vi "BRig_RT__Case_Exp__State_initTrial__v17.vi"(0 "input_dataCurrent":u16[](array[numeric]), 9 "input_dataBlock":u16[][](array[numeric]), 11 "input_dataTrial":u16[][](array[numeric]), 12 "input_dataExp":u16[](array[numeric])) -> (1 "output_iTrial":u16, 2 "output_nTrial":u16, 3 "output_SolenoidReward":bool, 4 "output_dataCurrent":u16[](array[numeric]), 10 "output_dataBlock":u16[][](array[numeric]), 15 "output_dataTrial":u16[][](array[numeric]))   [LabVIEW 2014]
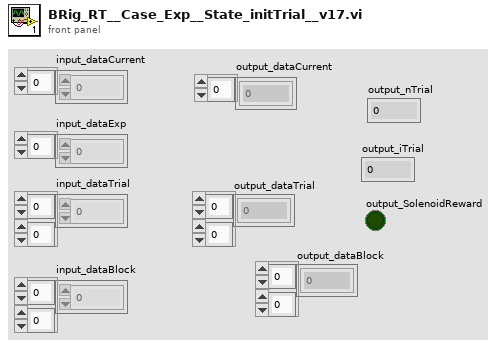
[diagram p1: front panel]
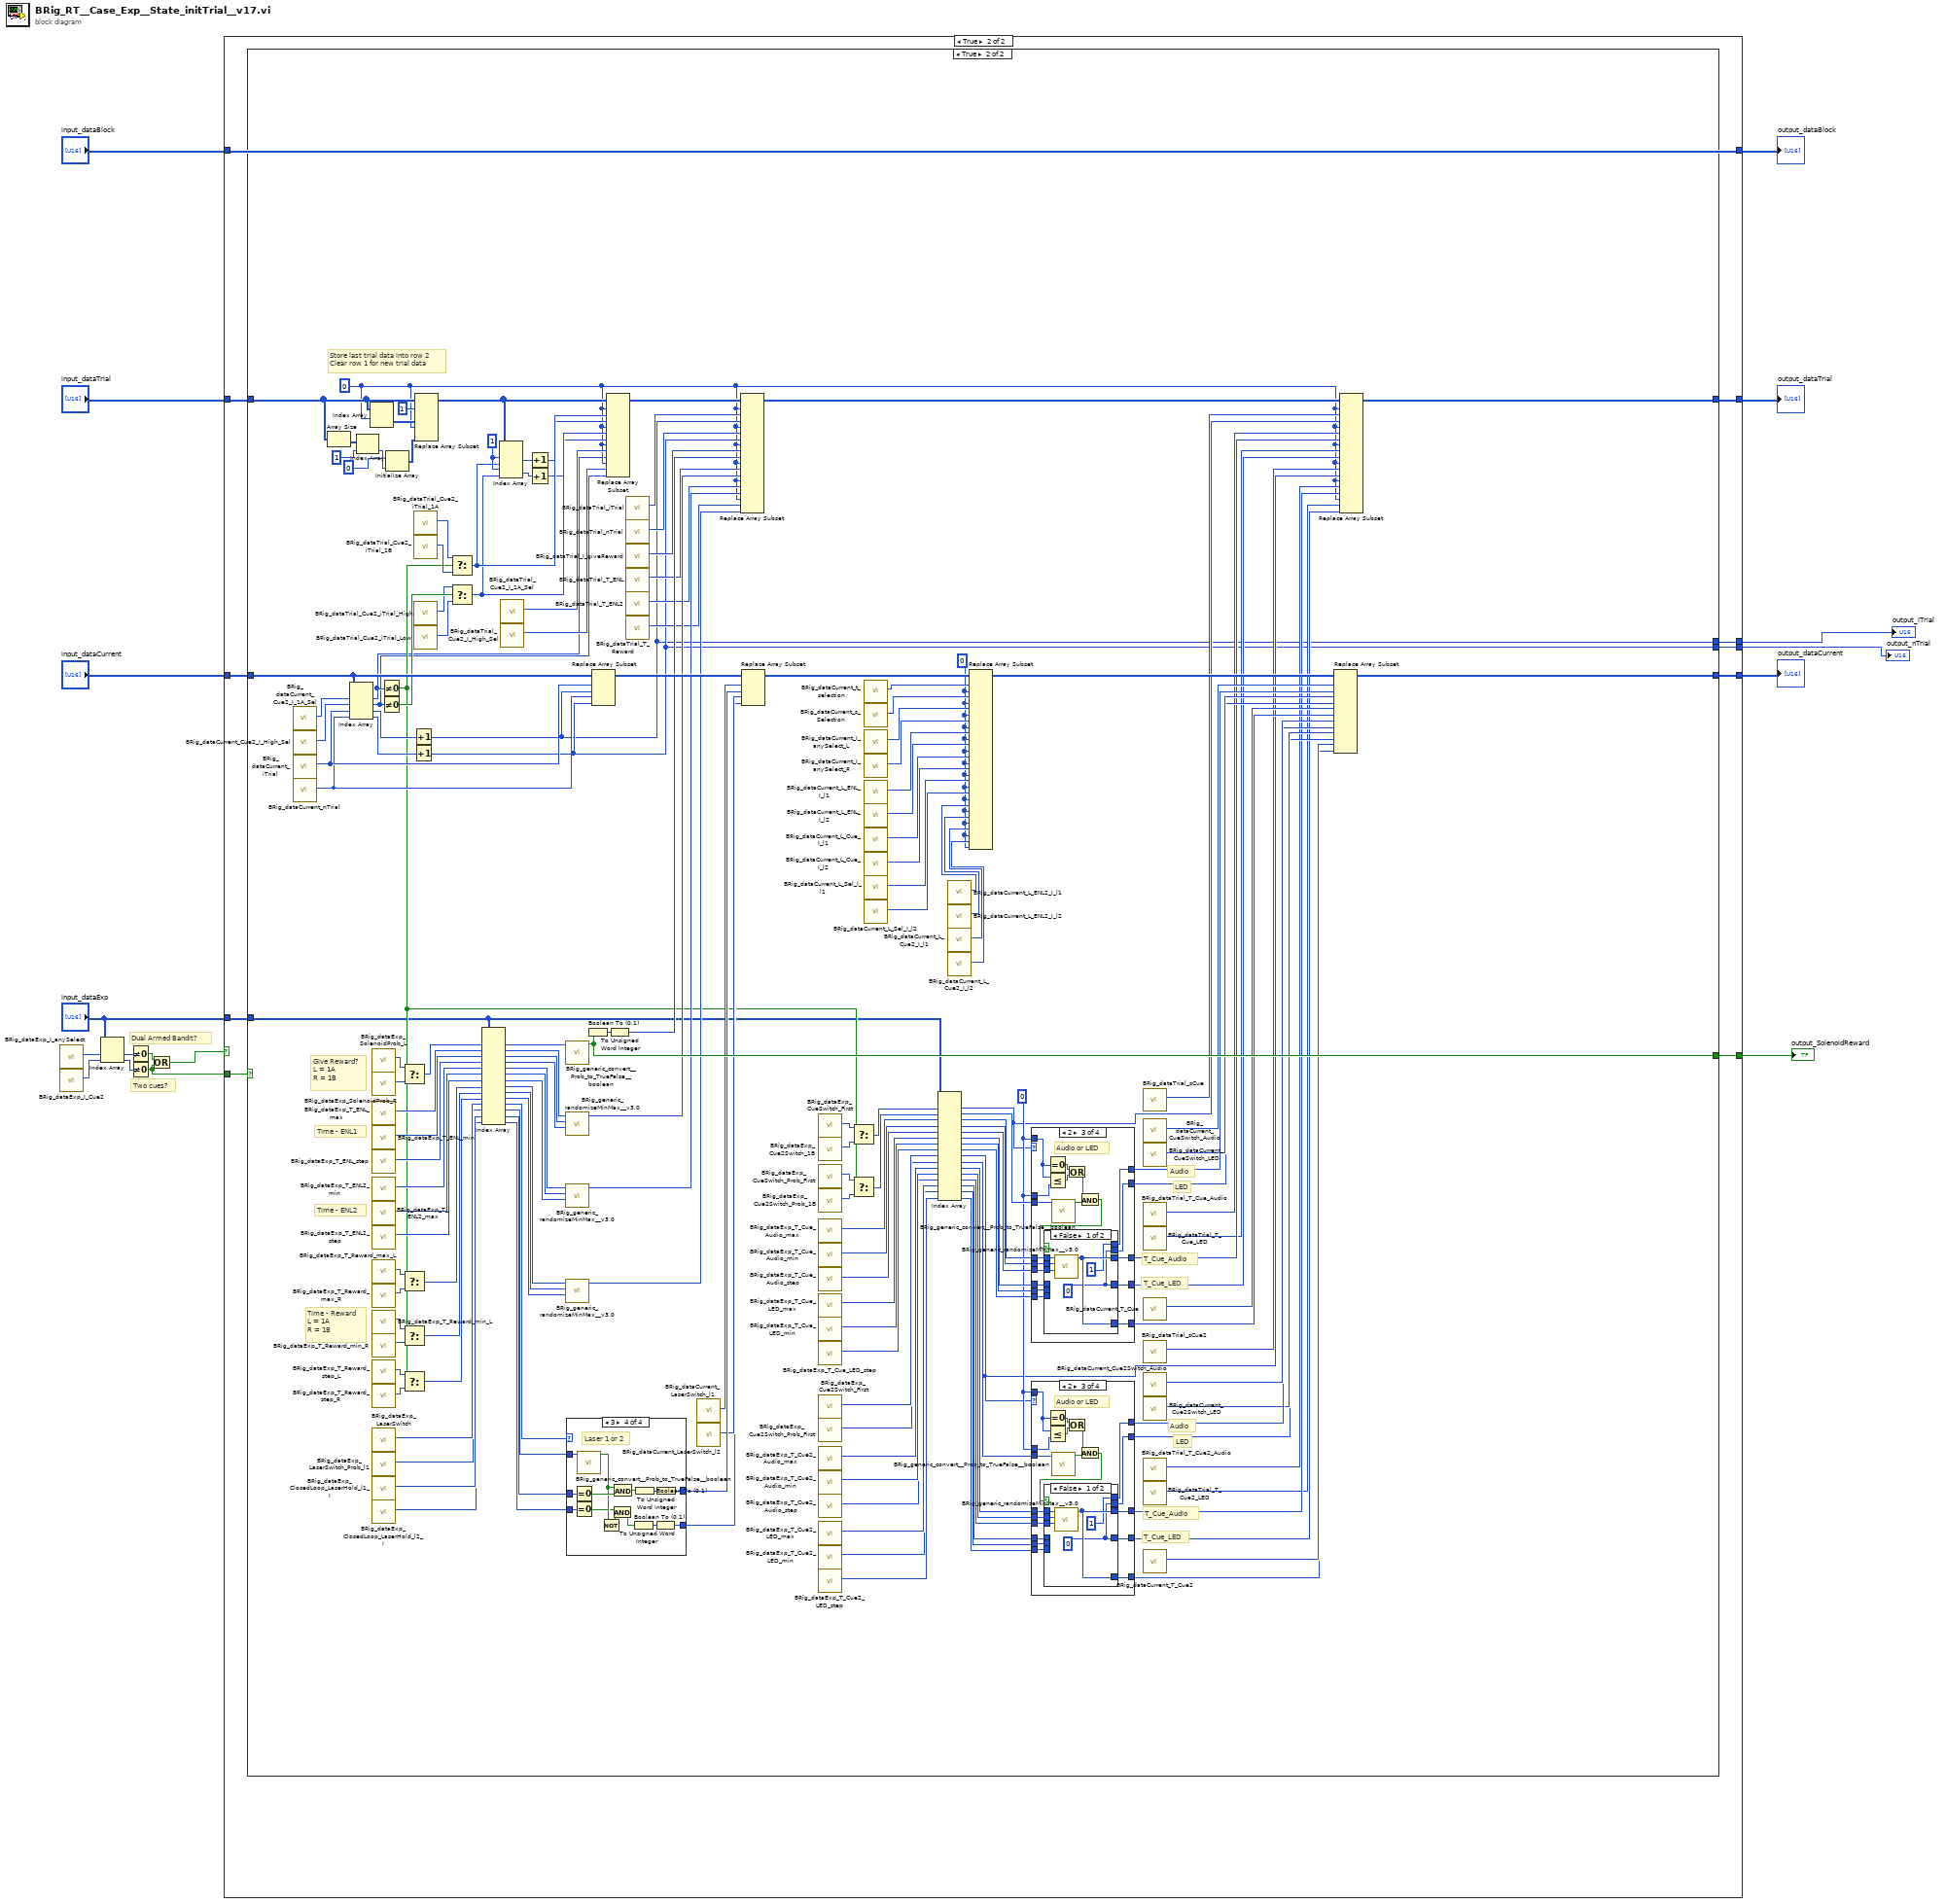
[diagram p0: block diagram]
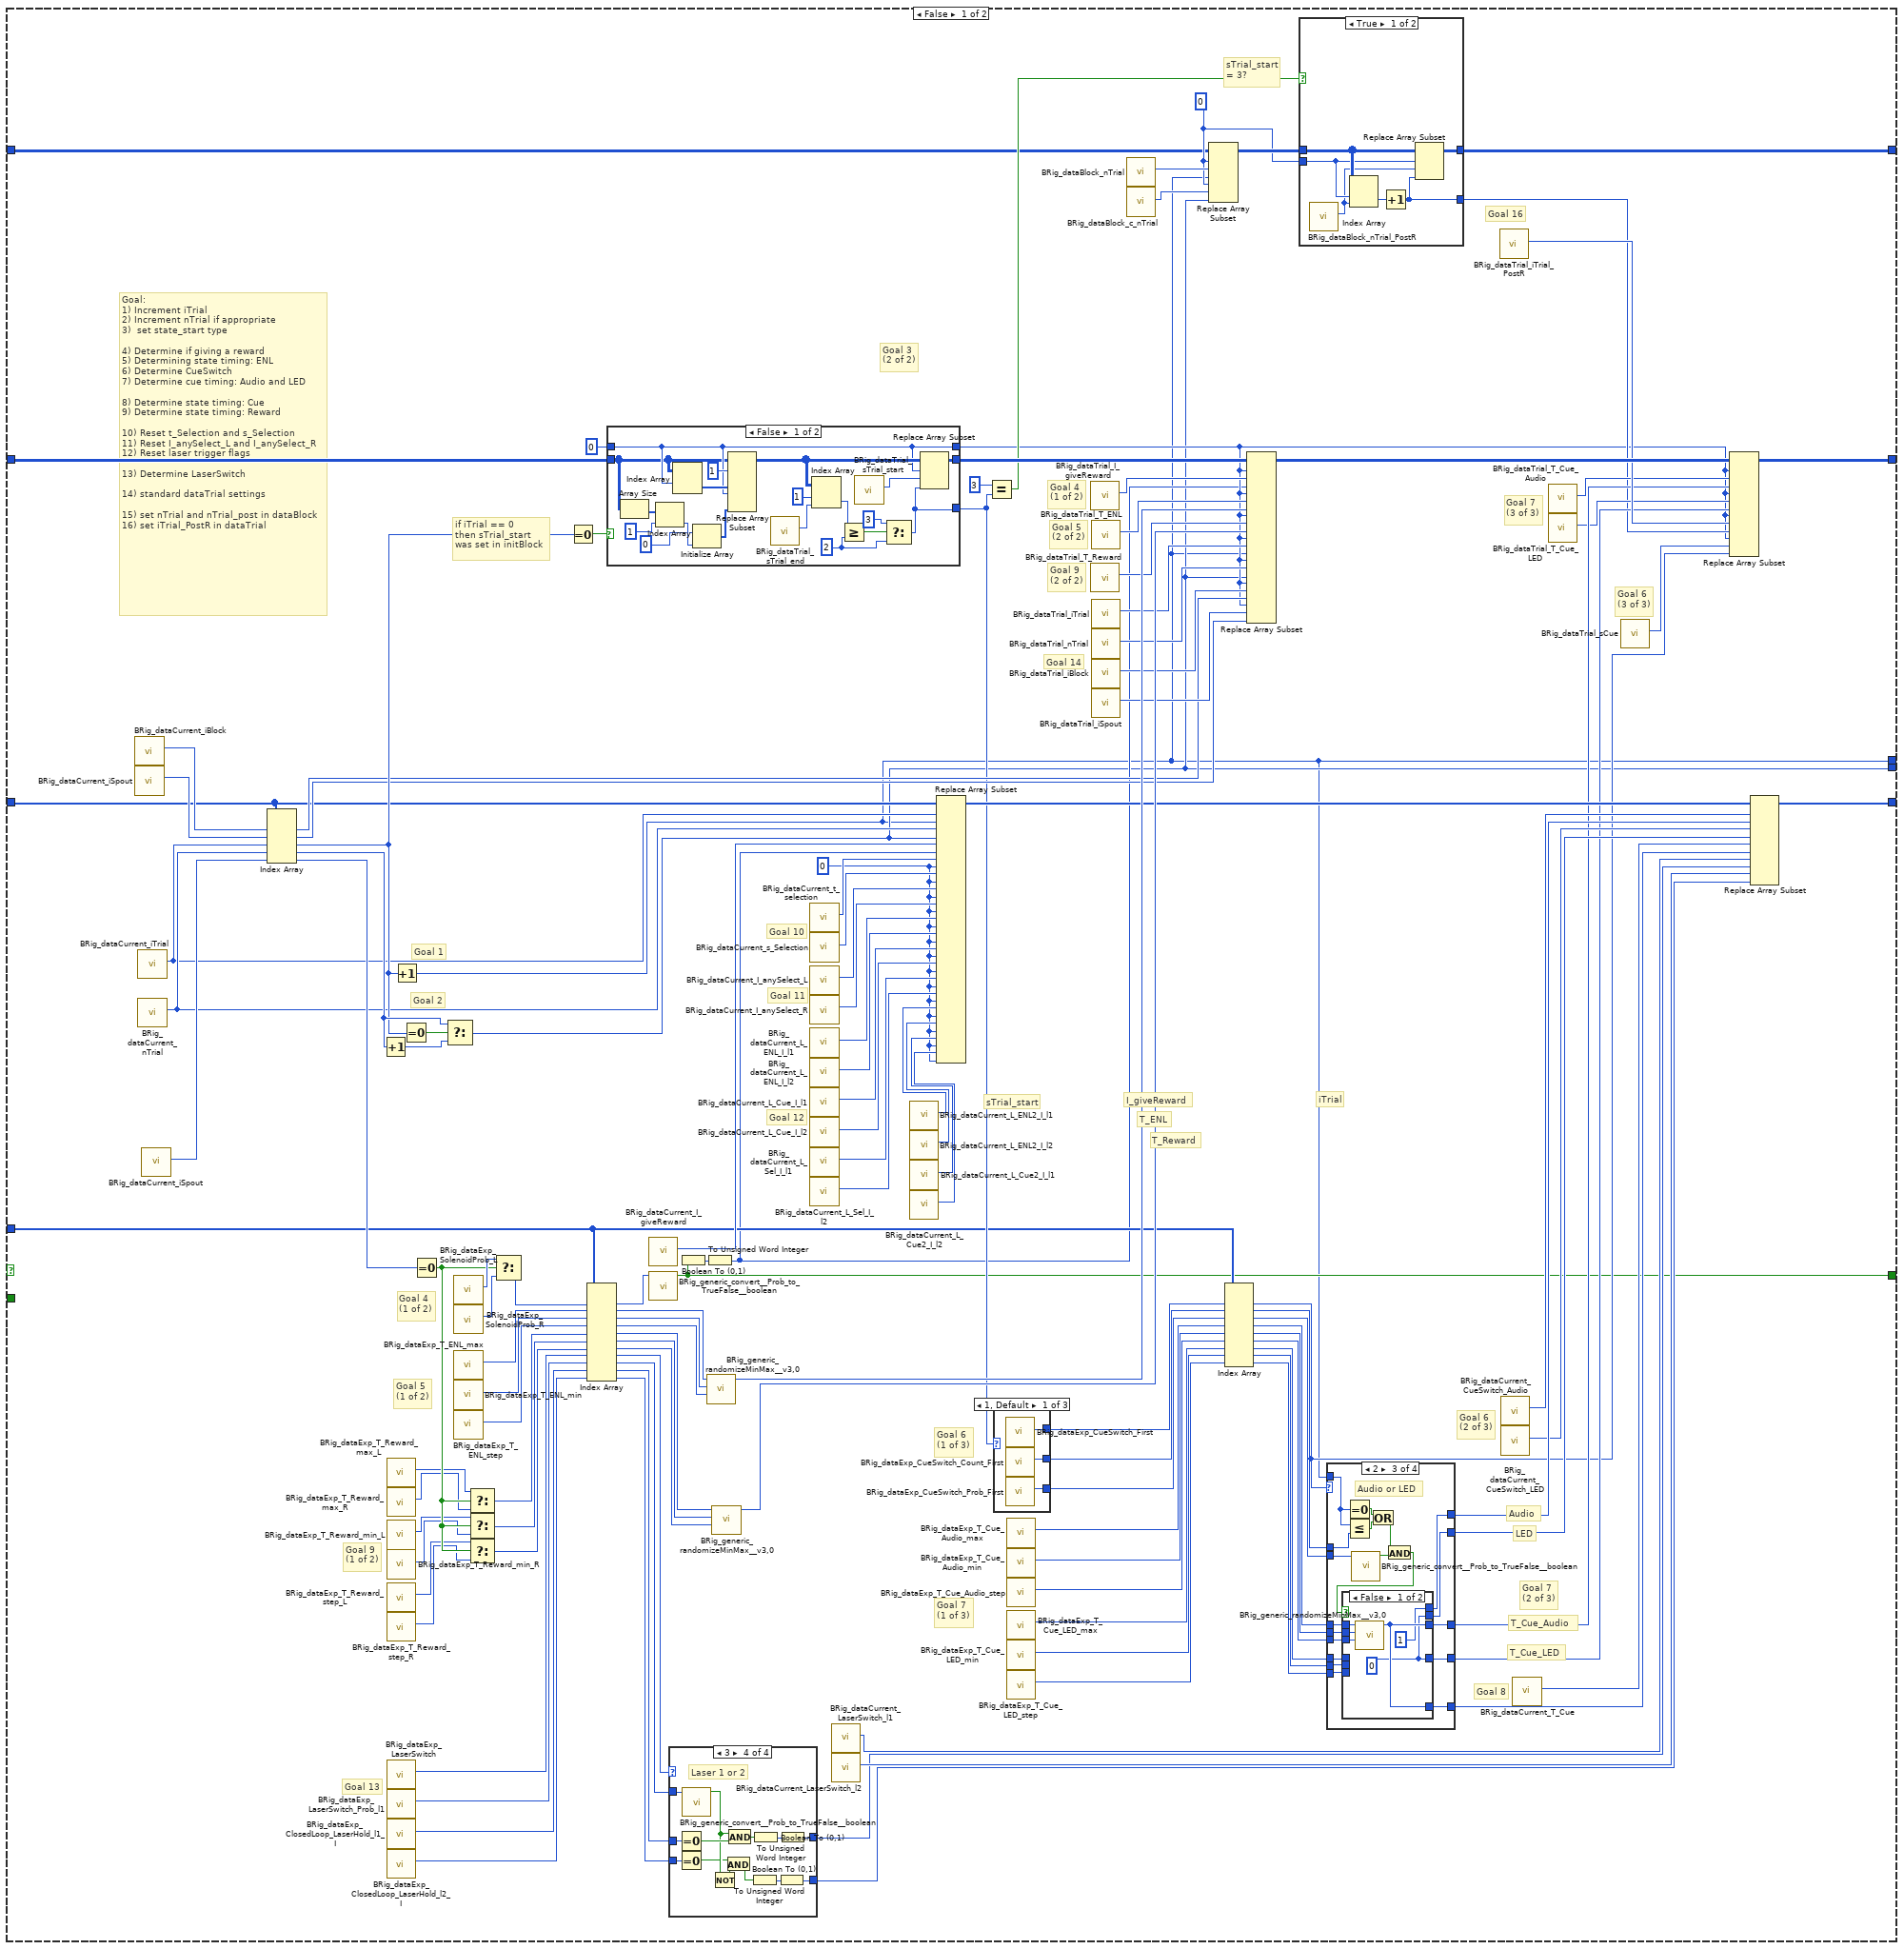
[diagram p2: hidden frame]
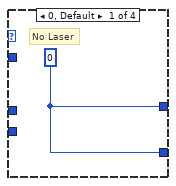
[diagram p4: hidden frame]
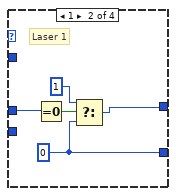
[diagram p5: hidden frame]
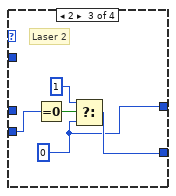
[diagram p6: hidden frame]
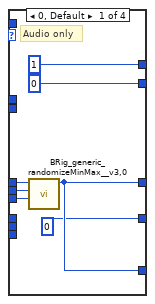
[diagram p7: hidden frame]
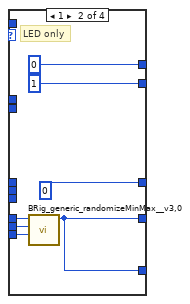
[diagram p8: hidden frame]
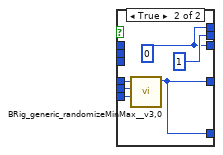
[diagram p9: hidden frame]
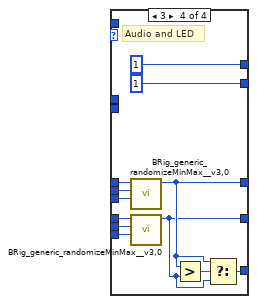
[diagram p10: hidden frame]
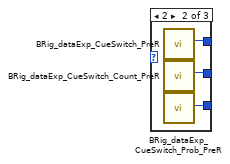
[diagram p11: hidden frame]
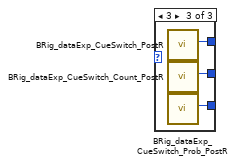
[diagram p12: hidden frame]
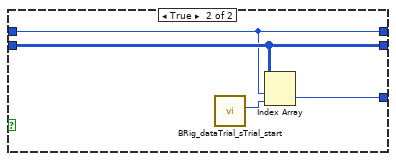
[diagram p13: hidden frame]
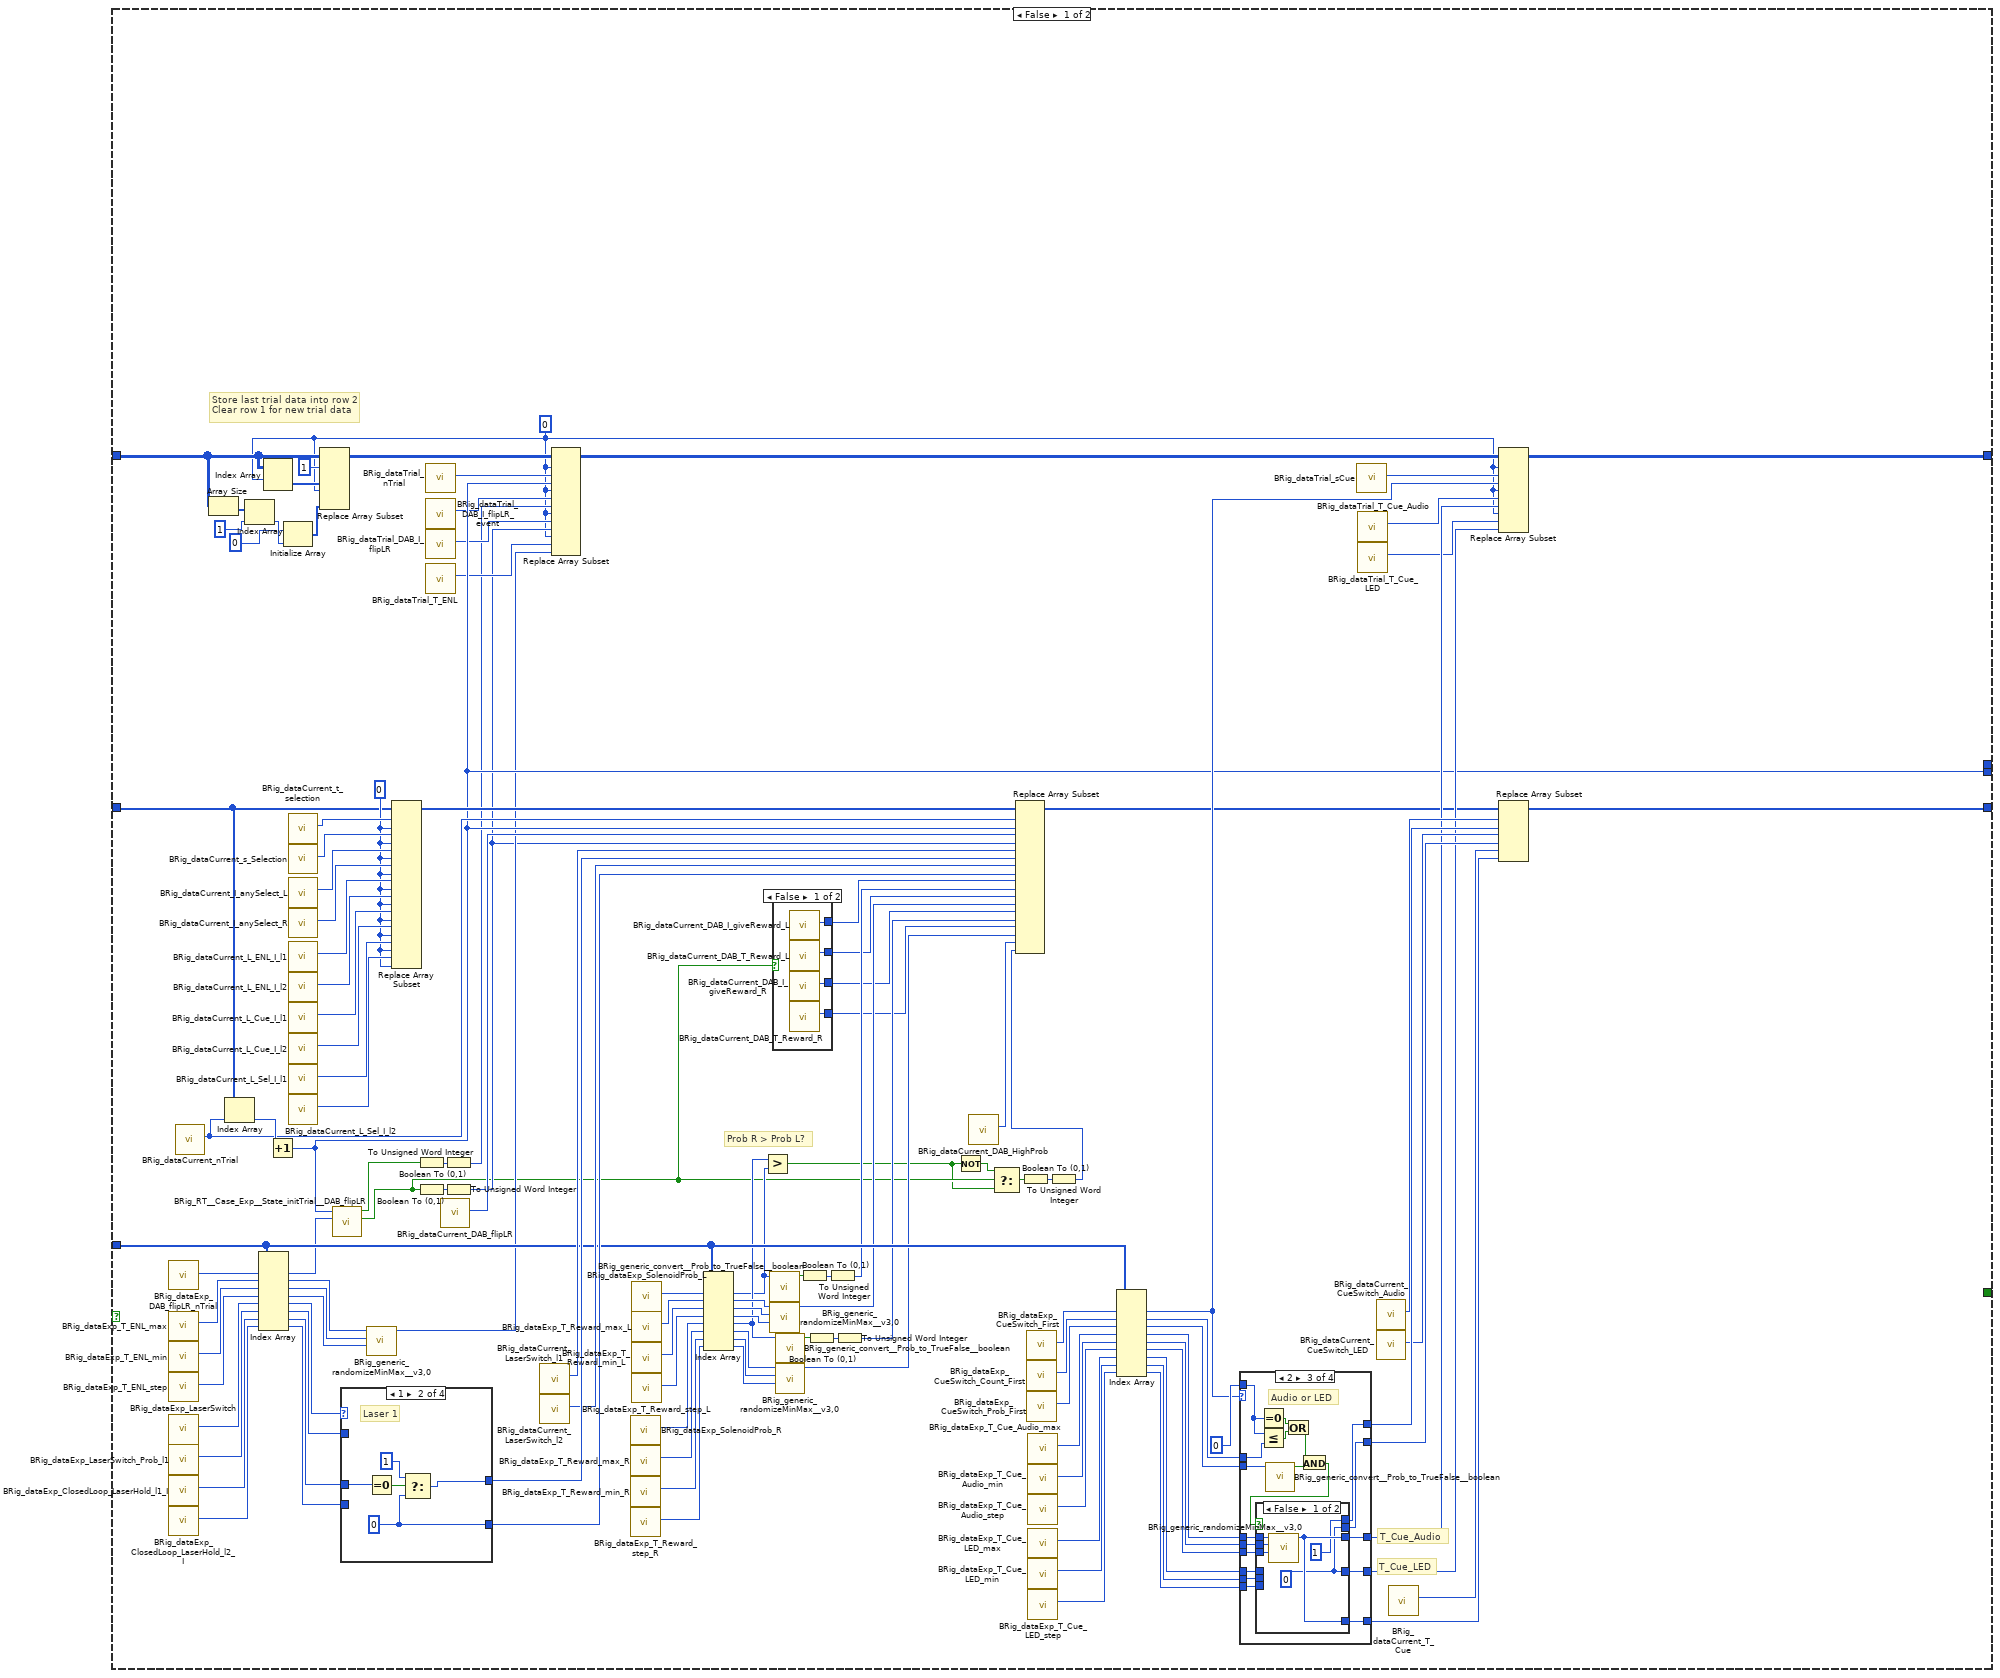
[diagram p14: hidden frame]
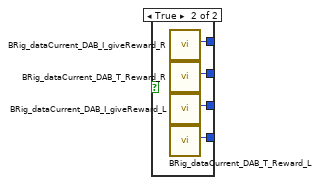
[diagram p15: hidden frame]
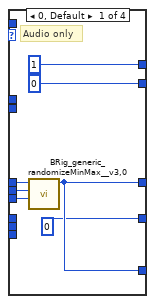
[diagram p16: hidden frame]
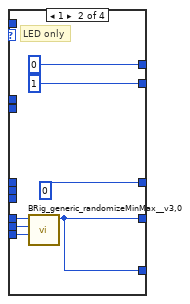
[diagram p17: hidden frame]
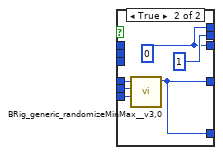
[diagram p18: hidden frame]
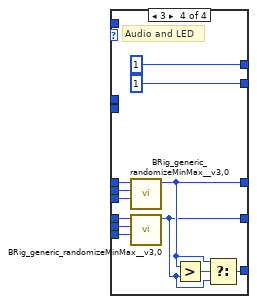
[diagram p19: hidden frame]
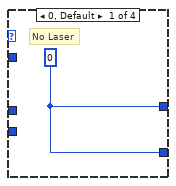
[diagram p20: hidden frame]
diagram:
  # "Two cues?"
  # "Dual Armed Bandit?"
  n1 = call "BRig_dataExp_I_anySelect.vi"() -> ("output_I_anySelect"=w8:i32)  [unwired: 11 in]
  n2 = call "BRig_dataExp_I_Cue2.vi"() -> ("output_I_Cue2"=w6:i32)  [unwired: 11 in]
  n3 = Index Array(array="input_dataExp", index #1=w8, index #2=w6) -> (element #1=w7:u16, element #2=w5:u16)
  n4 = Not Equal To 0?(x=w7) -> (x != 0?=w4:bool)
  n5 = Not Equal To 0?(x=w5) -> (x != 0?=w1:bool)
  n6 = Or(x=w4, y=w1) -> (x .or. y?=w2:bool)
  n7 = case shown="True" w2 {
    tunnel: "input_dataExp" -> [w28 w271]
    tunnel: "input_dataCurrent" -> [w27 w272]
    tunnel: "input_dataTrial" -> [w26 w269]
    tunnel: "input_dataBlock" -> [w25 w275]
    tunnel: [w24 w275] -> w14
    tunnel: [w23 w273] -> w13
    tunnel: [w22 w274] -> w12
    tunnel: [w21 w267] -> w11
    tunnel: [w19 w270] -> w10
    tunnel: [w18 w266] -> w9
    tunnel: w1 -> [_ w268]
    frame False {
      w39 = 0 ("disabled index (row)")
      w31 = u16 0 ("new element/subarray")
      # "Goal 16"
      # "Goal 6\n(3 of 3)"
      # "sTrial_start\n= 3?"
      # "Goal 14"
      # "Goal 13"
      # "iTrial"
      # "Goal 8"
      # "Goal 7\n(3 of 3)"
      # "Goal 7\n(2 of 3)"
      # "Goal 7\n(1 of 3)"
      # "T_Cue_LED"
      # "T_Cue_Audio"
      # "I_giveReward"
      # "Goal 4\n(1 of 2)"
      # "T_Reward"
      # "Goal 9\n(2 of 2)"
      # "Goal 9\n(1 of 2)"
      # "Goal 12"
      # "Goal 11"
      # "Goal 10"
      # "T_ENL"
      # "sTrial_start"
      # "LED"
      # "Audio"
      # "Goal 6\n(2 of 3)"
      # "Goal 6\n(1 of 3)"
      # "Goal 3\n(2 of 2)"
      # "Goal 5\n(2 of 2)"
      # "Goal 5\n(1 of 2)"
      # "Goal 4\n(1 of 2)"
      # "if iTrial == 0\nthen sTrial_start\nwas set in initBlock"
      # "Goal 2"
      # "Goal 1"
      # "Goal:\n1) Increment iTrial\n2) Increment nTrial if appropriate\n3)  set state_start type\n\n4) Determine if giving a reward\n5) Determining state timing: ENL\n6) Determine CueSwitch\n7) Determine cue timing: Audio and LED\n\n8) Determine state timing: Cue\n9) Determine state timing: Reward\n\n10) Reset t_Selection and s_Selection\n11) Reset I_anySelect_L and I_anySelect_R\n12) Reset laser trigger flags\n\n13) Determine LaserSwitch\n\n14) standard dataTrial settings\n\n15) set nTrial and nTrial_post in dataBlock\n16) set iTrial_PostR in dataTrial"
      n8 = call "BRig_dataCurrent_iBlock.vi"() -> ("output_iBlock"=w55:i32)  [unwired: 11 in]
      n9 = call "BRig_dataCurrent_iSpout.vi"() -> ("output_iSpout"=w54:i32)  [unwired: 11 in]
      n10 = call "BRig_dataCurrent_iTrial.vi"() -> ("output_iTrial"=w36:i32)  [unwired: 11 in]
      n11 = call "BRig_dataCurrent_nTrial.vi"() -> ("output_nTrial"=w37:i32)  [unwired: 11 in]
      n12 = call "BRig_dataCurrent_iSpout.vi"() -> ("output_iSpout"=w46:i32)  [unwired: 11 in]
      n13 = Index Array(array=w27, index #1=w55, index #2=w54, index #3=w36, index #4=w37, index #5=w46) -> (element #1=w64:u16, element #2=w63:u16, element #3=w77:u16, element #4=w144:u16, element #5=w45:u16)
      n14 = Increment(x=w144) -> (x+1=w143:u16)
      n15 = call "BRig_dataExp_T_Reward_max_L.vi"() -> ("output_T_Reward_max_L"=w108:i32)  [unwired: 11 in]
      n16 = call "BRig_dataExp_T_Reward_max_R.vi"() -> ("output_T_Reward_max_R"=w107:i32)  [unwired: 11 in]
      n17 = call "BRig_dataExp_T_Reward_min_L.vi"() -> ("output_Tcycle_Reward_min_L"=w106:i32)  [unwired: 11 in]
      n18 = call "BRig_dataExp_T_Reward_min_R.vi"() -> ("output_T_Reward_min_R"=w105:i32)  [unwired: 11 in]
      n19 = call "BRig_dataExp_T_Reward_step_L.vi"() -> ("output_T_Reward_step_L"=w104:i32)  [unwired: 11 in]
      n20 = call "BRig_dataExp_T_Reward_step_R.vi"() -> ("output_T_Reward_step_R"=w103:i32)  [unwired: 11 in]
      n21 = call "BRig_dataExp_LaserSwitch.vi"() -> ("output_LaserSwitch"=w76:i32)  [unwired: 11 in]
      n22 = call "BRig_dataExp_LaserSwitch_Prob_l1.vi"() -> ("output_LaserSwitch_Probability_L1"=w75:i32)  [unwired: 11 in]
      n23 = call "BRig_dataExp_ClosedLoop_LaserHold_l1_I.vi"() -> ("output_CloseLoop_LaserHold_l1_I"=w51:i32)  [unwired: 11 in]
      n24 = call "BRig_dataExp_ClosedLoop_LaserHold_l2_I.vi"() -> ("output_CloseLoop_LaserHold_l2_I"=w50:i32)  [unwired: 11 in]
      n25 = Increment(x=w77) -> (x+1=w18:u16)
      n26 = Equal To 0?(x=w77) -> (x = 0?=w142:bool)
      n27 = Equal To 0?(x=w45) -> (x = 0?=w109:bool)
      n28 = Select(t=w144, s=w142, f=w143) -> (s? t:f=w19:u16)
      n29 = call "BRig_dataExp_SolenoidProb_L.vi"() -> ("output_SolenoidProbability_L"=w139:i32)  [unwired: 11 in]
      n30 = call "BRig_dataExp_SolenoidProb_R.vi"() -> ("output_SolenoidProbability_R"=w138:i32)  [unwired: 11 in]
      n31 = call "BRig_dataExp_T_ENL_max.vi"() -> ("output_T_ENL_max"=w133:i32)  [unwired: 11 in]
      n32 = call "BRig_dataExp_T_ENL_min.vi"() -> ("output_T_ENL_min"=w134:i32)  [unwired: 11 in]
      n33 = call "BRig_dataExp_T_ENL_step.vi"() -> ("output_T_ENL_step"=w135:i32)  [unwired: 11 in]
      n34 = Select(t=w108, s=w109, f=w107) -> (s? t:f=w102:i32)
      n35 = Select(t=w106, s=w109, f=w105) -> (s? t:f=w101:i32)
      n36 = Select(t=w104, s=w109, f=w103) -> (s? t:f=w100:i32)
      n37 = Select(t=w139, s=w109, f=w138) -> (s? t:f=w137:i32)
      n38 = Equal To 0?(x=w77) -> (x = 0?=w141:bool)
      n39 = Index Array(array=w28, index #1=w137, index #2=w133, index #3=w134, index #4=w135, index #5=w102, index #6=w101, index #7=w100, index #8=w76, index #9=w75, index #10=w51, index #11=w50) -> (element #1=w136:u16, element #2=w132:u16, element #3=w131:u16, element #4=w130:u16, element #5=w99:u16, element #6=w98:u16, element #7=w97:u16, element #8=w74:u16, element #9=w73:u16, element #10=w49:u16, element #11=w48:u16)
      n40 = case shown="False" w141 {
        tunnel: w26 -> [w248 w265]
        tunnel: [w259 w265] -> w129
        tunnel: 0 -> [w249 w264]
        tunnel: [w249 w264] -> w29
        tunnel: [w255 w262] -> w30
        frame False {
          w256 = u16 2 ("y")
          n41 = Array Size(array=w248) -> (size(s)=w247:i32[])
          n42 = Index Array(array=w247, index=1) -> (element=w245:i32)
          n43 = Index Array(array=w248, index (row)=w249) -> (element=w252:u16[])  [unwired: 1 in]
          n44 = Initialize Array(u16 0 ("index"), w245) -> (w243:u16[])
          n45 = Replace Array Subset(array=w248, new element #1=w252, index (row) #1=1 ("index (row)"), new element #2=w243, index (row) #2=w249) -> (w250:u16[][])  [unwired: 2 in]
          n46 = call "BRig_dataTrial_sTrial_end.vi"() -> ("output_sTrial_end"=w261:i32)  [unwired: 11 in]
          n47 = Index Array(array=w250, index (row)=1 ("disabled index (row)"), index (col)=w261) -> (element=w260:u16)
          n48 = Greater Or Equal?(x=w260, y=w256) -> (x >= y?=w258:bool)
          n49 = call "BRig_dataTrial_sTrial_start.vi"() -> ("output_sTrial_start"=w254:i32)  [unwired: 11 in]
          n50 = Select(t=u16 3 ("y"), s=w258, f=w256) -> (s? t:f=w255:u16)
          n51 = Replace Array Subset(array=w250, new element=w255, index (row)=w249, index (col)=w254) -> (w259:u16[][])
        }
        frame True {
          n52 = call "BRig_dataTrial_sTrial_start.vi"() -> ("output_sTrial_start"=w263:i32)  [unwired: 11 in]
          n53 = Index Array(array=w265, index (row)=w264, index (col)=w263) -> (element=w262:u16)
        }
      }
      n54 = call "BRig_dataCurrent_I_giveReward.vi"() -> ("output_I_giveReward"=w140:i32)  [unwired: 11 in]
      n55 = call "BRig_generic_convert__Prob_to_TrueFalse__boolean.vi"("input_probability_u16"=w136) -> ("output_TF"=w21:bool)  [unwired: 10 in]
      n56 = case shown="3" w74 {
        tunnel: [w153 w154 w159 w173] -> w71
        tunnel: [w153 w155 w160 w172] -> w70
        tunnel: w73 -> [_ _ _ w176]
        tunnel: w49 -> [_ w158 _ w171]
        tunnel: w48 -> [_ _ w161 w170]
        frame 0, Default {
          w153 = u16 0
          # "No Laser"
        }
        frame 1 {
          w155 = u16 0
          # "Laser 1"
          n57 = Equal To 0?(x=w158) -> (x = 0?=w157:bool)
          n58 = Select(t=u16 1, s=w157, f=w155) -> (s? t:f=w154:u16)
        }
        frame 2 {
          w159 = u16 0
          # "Laser 2"
          n59 = Equal To 0?(x=w161) -> (x = 0?=w163:bool)
          n60 = Select(t=u16 1, s=w163, f=w159) -> (s? t:f=w160:u16)
        }
        frame 3 {
          # "Laser 1 or 2"
          n61 = Equal To 0?(x=w171) -> (x = 0?=w169:bool)
          n62 = Equal To 0?(x=w170) -> (x = 0?=w165:bool)
          n63 = call "BRig_generic_convert__Prob_to_TrueFalse__boolean.vi"("input_probability_u16"=w176) -> ("output_TF"=w168:bool)  [unwired: 10 in]
          n64 = Not(x=w168) -> (.not. x?=w166:bool)
          n65 = And(x=w165, y=w166) -> (x .and. y?=w164:bool)
          n66 = And(x=w168, y=w169) -> (x .and. y?=w167:bool)
          n67 = Boolean To (0,1)(Boolean=w164) -> (0, 1=w175:i16)
          n68 = Boolean To (0,1)(Boolean=w167) -> (0, 1=w174:i16)
          n69 = To Unsigned Word Integer(number=w175) -> (unsigned 16bit integer=w172:u16)
          n70 = To Unsigned Word Integer(number=w174) -> (unsigned 16bit integer=w173:u16)
        }
      }
      n71 = Boolean To (0,1)(Boolean=w21) -> (0, 1=w145:i16)
      n72 = To Unsigned Word Integer(number=w145) -> (unsigned 16bit integer=w20:u16)
      n73 = call "BRig_generic_randomizeMinMax__v3,0.vi"("Input_Increment"=w130, "Input_Min"=w131, "Input_Max"=w132) -> ("Output"=w127:u16)  [unwired: 8 in]
      n74 = call "BRig_generic_randomizeMinMax__v3,0.vi"("Input_Increment"=w97, "Input_Min"=w98, "Input_Max"=w99) -> ("Output"=w95:u16)  [unwired: 8 in]
      n75 = call "BRig_dataCurrent_t_selection.vi"() -> ("output_t_selection"=w119:i32)  [unwired: 11 in]
      n76 = call "BRig_dataCurrent_s_Selection.vi"() -> ("output_s_Selection"=w118:i32)  [unwired: 11 in]
      n77 = call "BRig_dataCurrent_I_anySelect_L.vi"() -> ("output_IanySelect_L"=w117:i32)  [unwired: 11 in]
      n78 = call "BRig_dataCurrent_I_anySelect_R.vi"() -> ("output_IanySelect_R"=w116:i32)  [unwired: 11 in]
      n79 = call "BRig_dataCurrent_L_ENL_I_l1.vi"() -> ("output_L_ENL_I_l1"=w115:i32)  [unwired: 11 in]
      n80 = call "BRig_dataCurrent_L_ENL_I_l2.vi"() -> ("output_L_ENL_I_l2"=w114:i32)  [unwired: 11 in]
      n81 = call "BRig_dataCurrent_L_Cue_I_l1.vi"() -> ("output_L_Cue_I_l1"=w113:i32)  [unwired: 11 in]
      n82 = call "BRig_dataCurrent_L_Cue_I_l2.vi"() -> ("output_L_Cue_I_l2"=w112:i32)  [unwired: 11 in]
      n83 = call "BRig_dataCurrent_L_Sel_I_l1.vi"() -> ("output_L_Sel_I_l1"=w111:i32)  [unwired: 11 in]
      n84 = call "BRig_dataCurrent_L_Sel_I_l2.vi"() -> ("output_L_Sel_I_l2"=w110:i32)  [unwired: 11 in]
      n85 = call "BRig_dataCurrent_LaserSwitch_l1.vi"() -> ("output_LaserSwitch_l1"=w69:i32)  [unwired: 11 in]
      n86 = call "BRig_dataCurrent_LaserSwitch_l2.vi"() -> ("output_LaserSwitch_l2"=w72:i32)  [unwired: 11 in]
      n87 = call "BRig_dataCurrent_L_ENL2_I_l1.vi"() -> ("output_L_ENL2_I_l1"=w35:i32)  [unwired: 11 in]
      n88 = call "BRig_dataCurrent_L_ENL2_I_l2.vi"() -> ("output_L_ENL2_I_l2"=w34:i32)  [unwired: 11 in]
      n89 = call "BRig_dataCurrent_L_Cue2_I_l1.vi"() -> ("output_L_Cue2_I_l1"=w33:i32)  [unwired: 11 in]
      n90 = call "BRig_dataCurrent_L_Cue2_I_l2.vi"() -> ("output_L_Cue2_I_l2"=w32:i32)  [unwired: 11 in]
      n91 = Replace Array Subset(array=w27, new element #1=w18, index #1=w36, new element #2=w19, index #2=w37, new element #3=w20, index #3=w140, new element #4=w31, index #4=w119, new element #5=w31, index #5=w118, new element #6=w31, index #6=w117, new element #7=w31, index #7=w116, new element #8=w31, index #8=w115, new element #9=w31, index #9=w114, new element #10=w31, index #10=w113, new element #11=w31, index #11=w112, new element #12=w31, index #12=w111, new element #13=w31, index #13=w110, new element #14=w31, index #14=w35, new element #15=w31, index #15=w34, new element #16=w31, index #16=w33, new element #17=w31, index #17=w32) -> (w62:u16[])
      n92 = Equal?(x=u16 3 ("y"), y=w30) -> (x = y?=w40:bool)
      n93 = case shown="1, Default" w30 {
        tunnel: [w236 w237 w242] -> w126
        tunnel: [w235 w238 w241] -> w125
        tunnel: [w234 w239 w240] -> w124
        frame 1, Default {
          n94 = call "BRig_dataExp_CueSwitch_First.vi"() -> ("output_CueSwitch_First"=w236:i32)  [unwired: 11 in]
          n95 = call "BRig_dataExp_CueSwitch_Count_First.vi"() -> ("output_CueSwitch_Count_First"=w235:i32)  [unwired: 11 in]
          n96 = call "BRig_dataExp_CueSwitch_Prob_First.vi"() -> ("output_CueSwitch_Prob_First"=w234:i32)  [unwired: 11 in]
        }
        frame 2 {
          n97 = call "BRig_dataExp_CueSwitch_PreR.vi"() -> ("output_CueSwitch_PreR"=w237:i32)  [unwired: 11 in]
          n98 = call "BRig_dataExp_CueSwitch_Count_PreR.vi"() -> ("output_CueSwitch_Count_PreR"=w238:i32)  [unwired: 11 in]
          n99 = call "BRig_dataExp_CueSwitch_Prob_PreR.vi"() -> ("output_CueSwitch_Prob_PreR"=w239:i32)  [unwired: 11 in]
        }
        frame 3 {
          n100 = call "BRig_dataExp_CueSwitch_PostR.vi"() -> ("output_CueSwitch_PostR"=w242:i32)  [unwired: 11 in]
          n101 = call "BRig_dataExp_CueSwitch_Count_PostR.vi"() -> ("output_CueSwitch_Count_PostR"=w241:i32)  [unwired: 11 in]
          n102 = call "BRig_dataExp_CueSwitch_Prob_PostR.vi"() -> ("output_CueSwitch_Prob_PostR"=w240:i32)  [unwired: 11 in]
        }
      }
      n103 = call "BRig_dataExp_T_Cue_Audio_max.vi"() -> ("output_T_Cue_Audio_max"=w93:i32)  [unwired: 11 in]
      n104 = call "BRig_dataExp_T_Cue_Audio_min.vi"() -> ("output_T_Cue_Audio_min"=w92:i32)  [unwired: 11 in]
      n105 = call "BRig_dataExp_T_Cue_Audio_step.vi"() -> ("output_T_Cue_Audio_step"=w91:i32)  [unwired: 11 in]
      n106 = call "BRig_dataExp_T_Cue_LED_max.vi"() -> ("output_T_Cue_LED_max"=w90:i32)  [unwired: 11 in]
      n107 = call "BRig_dataExp_T_Cue_LED_min.vi"() -> ("output_T_Cue_LED_min"=w89:i32)  [unwired: 11 in]
      n108 = call "BRig_dataExp_T_Cue_LED_step.vi"() -> ("output_T_Cue_LED_step"=w88:i32)  [unwired: 11 in]
      n109 = call "BRig_dataTrial_I_giveReward.vi"() -> ("output_I_giveReward"=w94:i32)  [unwired: 11 in]
      n110 = call "BRig_dataTrial_T_Reward.vi"() -> ("output_T_Reward"=w96:i32)  [unwired: 11 in]
      n111 = call "BRig_dataTrial_T_ENL.vi"() -> ("output_T_ENL"=w128:i32)  [unwired: 11 in]
      n112 = call "BRig_dataTrial_iTrial.vi"() -> ("output_iTrial"=w68:i32)  [unwired: 11 in]
      n113 = call "BRig_dataTrial_nTrial.vi"() -> ("output_nTrial"=w67:i32)  [unwired: 11 in]
      n114 = call "BRig_dataTrial_iBlock.vi"() -> ("output_iBlock"=w66:i32)  [unwired: 11 in]
      n115 = call "BRig_dataTrial_iSpout.vi"() -> ("output_iSpout"=w65:i32)  [unwired: 11 in]
      n116 = call "BRig_dataBlock_nTrial.vi"() -> ("output_nTrial"=w42:i32)  [unwired: 11 in]
      n117 = call "BRig_dataBlock_c_nTrial.vi"() -> ("output_c_nTrial"=w41:i32)  [unwired: 11 in]
      n118 = Replace Array Subset(array=w25, new element #1=w18, index (row) #1=w39, index (col) #1=w42, new element #2=w19, index (row) #2=w39, index (col) #2=w41) -> (w43:u16[][])
      n119 = Index Array(array=w28, index #1=w126, index #2=w125, index #3=w124, index #4=w93, index #5=w92, index #6=w91, index #7=w90, index #8=w89, index #9=w88) -> (element #1=w52:u16, element #2=w87:u16, element #3=w86:u16, element #4=w85:u16, element #5=w84:u16, element #6=w83:u16, element #7=w82:u16, element #8=w81:u16, element #9=w80:u16)
      n120 = Replace Array Subset(array=w129, new element #1=w20, index (row) #1=w29, index (col) #1=w94, new element #2=w127, index (row) #2=w29, index (col) #2=w128, new element #3=w95, index (row) #3=w29, index (col) #3=w96, new element #4=w18, index (row) #4=w29, index (col) #4=w68, new element #5=w19, index (row) #5=w29, index (col) #5=w67, new element #6=w64, index (row) #6=w29, index (col) #6=w66, new element #7=w63, index (row) #7=w29, index (col) #7=w65) -> (w61:u16[][])
      n121 = case shown="True" w40 {
        tunnel: w43 -> [w151 w152]
        tunnel: [w149 w152] -> w24
        tunnel: [w146 _] -> w38
        tunnel: w39 -> [w148 _]
        frame True {
          n122 = call "BRig_dataBlock_nTrial_PostR.vi"() -> ("output_nTrial_PostR"=w147:i32)  [unwired: 11 in]
          n123 = Index Array(array=w151, index (row)=w148, index (col)=w147) -> (element=w150:u16)
          n124 = Increment(x=w150) -> (x+1=w146:u16)
          n125 = Replace Array Subset(array=w151, new element=w146, index (row)=w148, index (col)=w147) -> (w149:u16[][])
        }
        frame False {
        }
      }
      n126 = case shown="2" w52 {
        tunnel: [u16 1 u16 0 w195 u16 1] -> w122
        tunnel: [u16 0 u16 1 w194 u16 1] -> w120
        tunnel: w87 -> [_ _ w208 _]
        tunnel: w86 -> [_ _ w205 _]
        tunnel: w85 -> [w181 _ w201 w231]
        tunnel: w84 -> [w180 _ w200 w230]
        tunnel: w83 -> [w179 _ w199 w229]
        tunnel: w82 -> [_ w188 w193 w228]
        tunnel: w81 -> [_ w187 w192 w227]
        tunnel: w80 -> [_ w186 w191 w226]
        tunnel: [w178 u16 0 ("Output") w198 w224] -> w59
        tunnel: [u16 0 ("Output") w185 w196 w223] -> w58
        tunnel: [w178 w185 w197 w222] -> w78
        tunnel: w18 -> [_ _ w209 _]
        frame 0, Default {
          # "Audio only"
          n127 = call "BRig_generic_randomizeMinMax__v3,0.vi"("Input_Increment"=w179, "Input_Min"=w180, "Input_Max"=w181) -> ("Output"=w178:u16)  [unwired: 8 in]
        }
        frame 1 {
          # "LED only"
          n128 = call "BRig_generic_randomizeMinMax__v3,0.vi"("Input_Increment"=w186, "Input_Min"=w187, "Input_Max"=w188) -> ("Output"=w185:u16)  [unwired: 8 in]
        }
        frame 2 {
          # "Audio or LED"
          n129 = Equal To 0?(x=w209) -> (x = 0?=w207:bool)
          n130 = Less Or Equal?(x=w209, y=w208) -> (x <= y?=w206:bool)
          n131 = call "BRig_generic_convert__Prob_to_TrueFalse__boolean.vi"("input_probability_u16"=w205) -> ("output_TF"=w204:bool)  [unwired: 10 in]
          n132 = Or(x=w207, y=w206) -> (x .or. y?=w203:bool)
          n133 = And(x=w203, y=w204) -> (x .and. y?=w202:bool)
          n134 = case shown="False" w202 {
            tunnel: w201 -> [w215 _]
            tunnel: w200 -> [w214 _]
            tunnel: w199 -> [w213 _]
            tunnel: [w212 w216] -> w198
            tunnel: [w212 w218] -> w197
            tunnel: [w210 w218] -> w196
            tunnel: [u16 1 w216] -> w195
            tunnel: [w210 u16 1] -> w194
            tunnel: w193 -> [_ w221]
            tunnel: w192 -> [_ w220]
            tunnel: w191 -> [_ w219]
            frame False {
              w210 = u16 0
              n135 = call "BRig_generic_randomizeMinMax__v3,0.vi"("Input_Increment"=w213, "Input_Min"=w214, "Input_Max"=w215) -> ("Output"=w212:u16)  [unwired: 8 in]
            }
            frame True {
              w216 = u16 0
              n136 = call "BRig_generic_randomizeMinMax__v3,0.vi"("Input_Increment"=w219, "Input_Min"=w220, "Input_Max"=w221) -> ("Output"=w218:u16)  [unwired: 8 in]
            }
          }
        }
        frame 3 {
          # "Audio and LED"
          n137 = call "BRig_generic_randomizeMinMax__v3,0.vi"("Input_Increment"=w229, "Input_Min"=w230, "Input_Max"=w231) -> ("Output"=w224:u16)  [unwired: 8 in]
          n138 = call "BRig_generic_randomizeMinMax__v3,0.vi"("Input_Increment"=w226, "Input_Min"=w227, "Input_Max"=w228) -> ("Output"=w223:u16)  [unwired: 8 in]
          n139 = Greater?(x=w224, y=w223) -> (0:w225:bool)
          n140 = Select(t=w224, s=w225, f=w223) -> (s? t:f=w222:u16)
        }
      }
      n141 = call "BRig_dataTrial_iTrial_PostR.vi"() -> ("output_iTrial_PostR"=w60:i32)  [unwired: 11 in]
      n142 = call "BRig_dataCurrent_CueSwitch_Audio.vi"() -> ("output_CueSwitch_Audio"=w123:i32)  [unwired: 11 in]
      n143 = call "BRig_dataCurrent_CueSwitch_LED.vi"() -> ("output_CueSwitch_LED"=w121:i32)  [unwired: 11 in]
      n144 = call "BRig_dataCurrent_T_Cue.vi"() -> ("output_T_Cue"=w79:i32)  [unwired: 11 in]
      n145 = call "BRig_dataTrial_T_Cue_Audio.vi"() -> ("output_T_Cue_Audio"=w57:i32)  [unwired: 11 in]
      n146 = call "BRig_dataTrial_T_Cue_LED.vi"() -> ("output_T_Cue_LED"=w56:i32)  [unwired: 11 in]
      n147 = call "BRig_dataTrial_sCue.vi"() -> ("output_sCue"=w53:i32)  [unwired: 11 in]
      n148 = Replace Array Subset(array=w61, new element #1=w59, index (row) #1=w29, index (col) #1=w57, new element #2=w58, index (row) #2=w29, index (col) #2=w56, new element #3=w38, index (row) #3=w29, index (col) #3=w60, new element #4=w52, index (row) #4=w29, index (col) #4=w53) -> (w23:u16[][])
      n149 = Replace Array Subset(array=w62, new element #1=w122, index #1=w123, new element #2=w120, index #2=w121, new element #3=w78, index #3=w79, new element #4=w71, index #4=w69, new element #5=w70, index #5=w72) -> (w22:u16[])
    }
    frame True {
      n150 = case shown="True" w268 {
        tunnel: [w356 w501] -> w274
        tunnel: [w355 w500] -> w273
        tunnel: w272 -> [w340 w660]
        tunnel: w271 -> [w331 w533]
        tunnel: [w305 w499] -> w270
        tunnel: w269 -> [w278 w649]
        tunnel: [_ w618] -> w267
        tunnel: [_ w498] -> w266
        frame False {
          w276 = 0
          w383 = u16 0 ("new element/subarray")
          # "Store last trial data into row 2\nClear row 1 for new trial data"
          # "Prob R > Prob L?"
          # "T_Cue_LED"
          # "T_Cue_Audio"
          n151 = call "BRig_dataExp_DAB_flipLR_nTrial.vi"() -> ("output_DAB_flipLR_nTrial"=w336:i32)  [unwired: 11 in]
          n152 = call "BRig_dataExp_T_ENL_max.vi"() -> ("output_T_ENL_max"=w400:i32)  [unwired: 11 in]
          n153 = call "BRig_dataExp_T_ENL_min.vi"() -> ("output_T_ENL_min"=w399:i32)  [unwired: 11 in]
          n154 = call "BRig_dataExp_T_ENL_step.vi"() -> ("output_T_ENL_step"=w398:i32)  [unwired: 11 in]
          n155 = call "BRig_dataExp_LaserSwitch.vi"() -> ("output_LaserSwitch"=w382:i32)  [unwired: 11 in]
          n156 = call "BRig_dataExp_LaserSwitch_Prob_l1.vi"() -> ("output_LaserSwitch_Probability_L1"=w381:i32)  [unwired: 11 in]
          n157 = call "BRig_dataExp_ClosedLoop_LaserHold_l1_I.vi"() -> ("output_CloseLoop_LaserHold_l1_I"=w380:i32)  [unwired: 11 in]
          n158 = call "BRig_dataExp_ClosedLoop_LaserHold_l2_I.vi"() -> ("output_CloseLoop_LaserHold_l2_I"=w379:i32)  [unwired: 11 in]
          n159 = call "BRig_dataCurrent_nTrial.vi"() -> ("output_nTrial"=w338:i32)  [unwired: 11 in]
          n160 = Array Size(array=w278) -> (size(s)=w283:i32[])
          n161 = Index Array(array=w340, index=w338) -> (element=w401:u16)
          n162 = Index Array(array=w283, index=1) -> (element=w281:i32)
          n163 = Index Array(array=w331, index #1=w336, index #2=w400, index #3=w399, index #4=w398, index #5=w382, index #6=w381, index #7=w380, index #8=w379) -> (element #1=w287:u16, element #2=w396:u16, element #3=w395:u16, element #4=w394:u16, element #5=w378:u16, element #6=w377:u16, element #7=w376:u16, element #8=w375:u16)
          n164 = Index Array(array=w278, index (row)=w276) -> (element=w285:u16[])  [unwired: 1 in]
          n165 = Increment(x=w401) -> (x+1=w305:u16)
          n166 = Initialize Array(u16 0 ("index"), w281) -> (w279:u16[])
          n167 = call "BRig_dataCurrent_t_selection.vi"() -> ("output_t_selection"=w393:i32)  [unwired: 11 in]
          n168 = call "BRig_dataCurrent_s_Selection.vi"() -> ("output_s_Selection"=w392:i32)  [unwired: 11 in]
          n169 = call "BRig_dataCurrent_I_anySelect_L.vi"() -> ("output_IanySelect_L"=w391:i32)  [unwired: 11 in]
          n170 = call "BRig_dataCurrent_I_anySelect_R.vi"() -> ("output_IanySelect_R"=w390:i32)  [unwired: 11 in]
          n171 = call "BRig_dataCurrent_L_ENL_I_l1.vi"() -> ("output_L_ENL_I_l1"=w389:i32)  [unwired: 11 in]
          n172 = call "BRig_dataCurrent_L_ENL_I_l2.vi"() -> ("output_L_ENL_I_l2"=w388:i32)  [unwired: 11 in]
          n173 = call "BRig_dataCurrent_L_Cue_I_l1.vi"() -> ("output_L_Cue_I_l1"=w387:i32)  [unwired: 11 in]
          n174 = call "BRig_dataCurrent_L_Cue_I_l2.vi"() -> ("output_L_Cue_I_l2"=w386:i32)  [unwired: 11 in]
          n175 = call "BRig_dataCurrent_L_Sel_I_l1.vi"() -> ("output_L_Sel_I_l1"=w385:i32)  [unwired: 11 in]
          n176 = call "BRig_dataCurrent_L_Sel_I_l2.vi"() -> ("output_L_Sel_I_l2"=w384:i32)  [unwired: 11 in]
          n177 = Replace Array Subset(array=w278, new element #1=w285, index (row) #1=1 ("index (row)"), new element #2=w279, index (row) #2=w276) -> (w277:u16[][])  [unwired: 2 in]
          n178 = call "BRig_RT__Case_Exp__State_initTrial__DAB_flipLR.vi"("input_DAB_flipLR_nTrial"=w287, "input_nTrial"=w305) -> ("output_switchedLR"=w293:bool, "output_flipOccurred"=w304:bool)  [unwired: 8 in]
          n179 = case shown="1" w378 {
            tunnel: [w467 w468 w473 w487] -> w334
            tunnel: [w467 w469 w474 w486] -> w332
            tunnel: w377 -> [_ _ _ w490]
            tunnel: w376 -> [_ w472 _ w485]
            tunnel: w375 -> [_ _ w475 w484]
            frame 0, Default {
              w467 = u16 0
              # "No Laser"
            }
            frame 1 {
              w469 = u16 0
              # "Laser 1"
              n180 = Equal To 0?(x=w472) -> (x = 0?=w471:bool)
              n181 = Select(t=u16 1, s=w471, f=w469) -> (s? t:f=w468:u16)
            }
            frame 2 {
              w473 = u16 0
              # "Laser 2"
              n182 = Equal To 0?(x=w475) -> (x = 0?=w477:bool)
              n183 = Select(t=u16 1, s=w477, f=w473) -> (s? t:f=w474:u16)
            }
            frame 3 {
              # "Laser 1 or 2"
              n184 = Equal To 0?(x=w485) -> (x = 0?=w483:bool)
              n185 = Equal To 0?(x=w484) -> (x = 0?=w479:bool)
              n186 = call "BRig_generic_convert__Prob_to_TrueFalse__boolean.vi"("input_probability_u16"=w490) -> ("output_TF"=w482:bool)  [unwired: 10 in]
              n187 = Not(x=w482) -> (.not. x?=w480:bool)
              n188 = And(x=w479, y=w480) -> (x .and. y?=w478:bool)
              n189 = And(x=w482, y=w483) -> (x .and. y?=w481:bool)
              n190 = Boolean To (0,1)(Boolean=w478) -> (0, 1=w489:i16)
              n191 = Boolean To (0,1)(Boolean=w481) -> (0, 1=w488:i16)
              n192 = To Unsigned Word Integer(number=w489) -> (unsigned 16bit integer=w486:u16)
              n193 = To Unsigned Word Integer(number=w488) -> (unsigned 16bit integer=w487:u16)
            }
          }
          n194 = call "BRig_generic_randomizeMinMax__v3,0.vi"("Input_Increment"=w394, "Input_Min"=w395, "Input_Max"=w396) -> ("Output"=w302:u16)  [unwired: 8 in]
          n195 = Replace Array Subset(array=w340, new element #1=w383, index #1=w393, new element #2=w383, index #2=w392, new element #3=w383, index #3=w391, new element #4=w383, index #4=w390, new element #5=w383, index #5=w389, new element #6=w383, index #6=w388, new element #7=w383, index #7=w387, new element #8=w383, index #8=w386, new element #9=w383, index #9=w385, new element #10=w383, index #10=w384) -> ()  [unwired: 1 out]
          n196 = Boolean To (0,1)(Boolean=w304) -> (0, 1=w306:i16)
          n197 = Boolean To (0,1)(Boolean=w293) -> (0, 1=w303:i16)
          n198 = call "BRig_dataTrial_nTrial.vi"() -> ("output_nTrial"=w341:i32)  [unwired: 11 in]
          n199 = call "BRig_dataTrial_DAB_I_flipLR_event.vi"() -> ("output_DAB_I_flipLR_event"=w300:i32)  [unwired: 11 in]
          n200 = call "BRig_dataTrial_DAB_I_flipLR.vi"() -> ("output_DAB_I_flipLR"=w299:i32)  [unwired: 11 in]
          n201 = call "BRig_dataTrial_T_ENL.vi"() -> ("output_T_ENL"=w301:i32)  [unwired: 11 in]
          n202 = call "BRig_dataCurrent_DAB_flipLR.vi"() -> ("output_DAB_flipLR"=w337:i32)  [unwired: 11 in]
          n203 = To Unsigned Word Integer(number=w306) -> (unsigned 16bit integer=w298:u16)
          n204 = To Unsigned Word Integer(number=w303) -> (unsigned 16bit integer=w297:u16)
          n205 = call "BRig_dataCurrent_LaserSwitch_l1.vi"() -> ("output_LaserSwitch_l1"=w335:i32)  [unwired: 11 in]
          n206 = call "BRig_dataCurrent_LaserSwitch_l2.vi"() -> ("output_LaserSwitch_l2"=w333:i32)  [unwired: 11 in]
          n207 = Replace Array Subset(array=w277, new element #1=w305, index (row) #1=w276, index (col) #1=w341, new element #2=w298, index (row) #2=w276, index (col) #2=w300, new element #3=w297, index (row) #3=w276, index (col) #3=w299, new element #4=w302, index (row) #4=w276, index (col) #4=w301) -> (w286:u16[][])
          n208 = call "BRig_dataExp_SolenoidProb_R.vi"() -> ("output_SolenoidProbability_R"=w326:i32)  [unwired: 11 in]
          n209 = call "BRig_dataExp_T_Reward_max_R.vi"() -> ("output_T_Reward_max_R"=w325:i32)  [unwired: 11 in]
          n210 = call "BRig_dataExp_T_Reward_min_R.vi"() -> ("output_T_Reward_min_R"=w324:i32)  [unwired: 11 in]
          n211 = call "BRig_dataExp_T_Reward_step_R.vi"() -> ("output_T_Reward_step_R"=w323:i32)  [unwired: 11 in]
          n212 = call "BRig_dataExp_SolenoidProb_L.vi"() -> ("output_SolenoidProbability_L"=w330:i32)  [unwired: 11 in]
          n213 = call "BRig_dataExp_T_Reward_max_L.vi"() -> ("output_T_Reward_max_L"=w329:i32)  [unwired: 11 in]
          n214 = call "BRig_dataExp_T_Reward_min_L.vi"() -> ("output_Tcycle_Reward_min_L"=w328:i32)  [unwired: 11 in]
          n215 = call "BRig_dataExp_T_Reward_step_L.vi"() -> ("output_T_Reward_step_L"=w327:i32)  [unwired: 11 in]
          n216 = Index Array(array=w331, index #1=w330, index #2=w329, index #3=w328, index #4=w327, index #5=w326, index #6=w325, index #7=w324, index #8=w323) -> (element #1=w295:u16, element #2=w322:u16, element #3=w321:u16, element #4=w320:u16, element #5=w296:u16, element #6=w319:u16, element #7=w318:u16, element #8=w317:u16)
          n217 = Greater?(x=w296, y=w295) -> (0:w292:bool)
          n218 = call "BRig_generic_convert__Prob_to_TrueFalse__boolean.vi"("input_probability_u16"=w295) -> ("output_TF"=w342:bool)  [unwired: 10 in]
          n219 = call "BRig_generic_randomizeMinMax__v3,0.vi"("Input_Increment"=w320, "Input_Min"=w321, "Input_Max"=w322) -> ("Output"=w311:u16)  [unwired: 8 in]
          n220 = case shown="False" w293 {
            tunnel: [w405 w408] -> w314
            tunnel: [w404 w407] -> w312
            tunnel: [w403 w406] -> w310
            tunnel: [w402 w409] -> w308
            frame False {
              n221 = call "BRig_dataCurrent_DAB_I_giveReward_L.vi"() -> ("output_DAB_I_giveReward_L"=w405:i32)  [unwired: 11 in]
              n222 = call "BRig_dataCurrent_DAB_T_Reward_L.vi"() -> ("output_DAB_T_Reward_L"=w404:i32)  [unwired: 11 in]
              n223 = call "BRig_dataCurrent_DAB_I_giveReward_R.vi"() -> ("output_DAB_I_giveReward_R"=w403:i32)  [unwired: 11 in]
              n224 = call "BRig_dataCurrent_DAB_T_Reward_R.vi"() -> ("output_DAB_T_Reward_R"=w402:i32)  [unwired: 11 in]
            }
            frame True {
              n225 = call "BRig_dataCurrent_DAB_I_giveReward_R.vi"() -> ("output_DAB_I_giveReward_R"=w408:i32)  [unwired: 11 in]
              n226 = call "BRig_dataCurrent_DAB_T_Reward_R.vi"() -> ("output_DAB_T_Reward_R"=w407:i32)  [unwired: 11 in]
              n227 = call "BRig_dataCurrent_DAB_I_giveReward_L.vi"() -> ("output_DAB_I_giveReward_L"=w406:i32)  [unwired: 11 in]
              n228 = call "BRig_dataCurrent_DAB_T_Reward_L.vi"() -> ("output_DAB_T_Reward_L"=w409:i32)  [unwired: 11 in]
            }
          }
          n229 = call "BRig_generic_convert__Prob_to_TrueFalse__boolean.vi"("input_probability_u16"=w296) -> ("output_TF"=w315:bool)  [unwired: 10 in]
          n230 = call "BRig_generic_randomizeMinMax__v3,0.vi"("Input_Increment"=w317, "Input_Min"=w318, "Input_Max"=w319) -> ("Output"=w307:u16)  [unwired: 8 in]
          n231 = Boolean To (0,1)(Boolean=w342) -> (0, 1=w397:i16)
          n232 = Boolean To (0,1)(Boolean=w315) -> (0, 1=w316:i16)
          n233 = To Unsigned Word Integer(number=w397) -> (unsigned 16bit integer=w313:u16)
          n234 = To Unsigned Word Integer(number=w316) -> (unsigned 16bit integer=w309:u16)
          n235 = Not(x=w292) -> (.not. x?=w294:bool)
          n236 = call "BRig_dataCurrent_DAB_HighProb.vi"() -> ("output_DAB_HighProb"=w289:i32)  [unwired: 11 in]
          n237 = Select(t=w294, s=w293, f=w292) -> (s? t:f=w290:bool)
          n238 = Boolean To (0,1)(Boolean=w290) -> (0, 1=w291:i16)
          n239 = call "BRig_dataExp_CueSwitch_First.vi"() -> ("output_CueSwitch_First"=w374:i32)  [unwired: 11 in]
          n240 = call "BRig_dataExp_CueSwitch_Count_First.vi"() -> ("output_CueSwitch_Count_First"=w373:i32)  [unwired: 11 in]
          n241 = call "BRig_dataExp_CueSwitch_Prob_First.vi"() -> ("output_CueSwitch_Prob_First"=w372:i32)  [unwired: 11 in]
          n242 = call "BRig_dataExp_T_Cue_Audio_max.vi"() -> ("output_T_Cue_Audio_max"=w371:i32)  [unwired: 11 in]
          n243 = call "BRig_dataExp_T_Cue_Audio_min.vi"() -> ("output_T_Cue_Audio_min"=w370:i32)  [unwired: 11 in]
          n244 = call "BRig_dataExp_T_Cue_Audio_step.vi"() -> ("output_T_Cue_Audio_step"=w369:i32)  [unwired: 11 in]
          n245 = call "BRig_dataExp_T_Cue_LED_max.vi"() -> ("output_T_Cue_LED_max"=w368:i32)  [unwired: 11 in]
          n246 = call "BRig_dataExp_T_Cue_LED_min.vi"() -> ("output_T_Cue_LED_min"=w367:i32)  [unwired: 11 in]
          n247 = call "BRig_dataExp_T_Cue_LED_step.vi"() -> ("output_T_Cue_LED_step"=w366:i32)  [unwired: 11 in]
          n248 = To Unsigned Word Integer(number=w291) -> (unsigned 16bit integer=w288:u16)
          n249 = Replace Array Subset(array=w340, new element #1=w305, index #1=w338, new element #2=w297, index #2=w337, new element #3=w334, index #3=w335, new element #4=w332, index #4=w333, new element #5=w313, index #5=w314, new element #6=w311, index #6=w312, new element #7=w309, index #7=w310, new element #8=w307, index #8=w308, new element #9=w288, index #9=w289) -> (w339:u16[])
          n250 = Index Array(array=w331, index #1=w374, index #2=w373, index #3=w372, index #4=w371, index #5=w370, index #6=w369, index #7=w368, index #8=w367, index #9=w366) -> (element #1=w349:u16, element #2=w364:u16, element #3=w363:u16, element #4=w362:u16, element #5=w361:u16, element #6=w360:u16, element #7=w359:u16, element #8=w358:u16, element #9=w357:u16)
          n251 = case shown="2" w349 {
            tunnel: [u16 1 u16 0 w428 u16 1] -> w353
            tunnel: [u16 0 u16 1 w427 u16 1] -> w351
            tunnel: w364 -> [_ _ w441 _]
            tunnel: w363 -> [_ _ w438 _]
            tunnel: w362 -> [w414 _ w434 w464]
            tunnel: w361 -> [w413 _ w433 w463]
            tunnel: w360 -> [w412 _ w432 w462]
            tunnel: w359 -> [_ w421 w426 w461]
            tunnel: w358 -> [_ w420 w425 w460]
            tunnel: w357 -> [_ w419 w424 w459]
            tunnel: [w411 u16 0 ("Output") w431 w457] -> w347
            tunnel: [u16 0 ("Output") w418 w429 w456] -> w345
            tunnel: [w411 w418 w430 w455] -> w343
            tunnel: u16 0 -> [_ _ w442 _]
            frame 0, Default {
              # "Audio only"
              n252 = call "BRig_generic_randomizeMinMax__v3,0.vi"("Input_Increment"=w412, "Input_Min"=w413, "Input_Max"=w414) -> ("Output"=w411:u16)  [unwired: 8 in]
            }
            frame 1 {
              # "LED only"
              n253 = call "BRig_generic_randomizeMinMax__v3,0.vi"("Input_Increment"=w419, "Input_Min"=w420, "Input_Max"=w421) -> ("Output"=w418:u16)  [unwired: 8 in]
            }
            frame 2 {
              # "Audio or LED"
              n254 = Equal To 0?(x=w442) -> (x = 0?=w440:bool)
              n255 = Less Or Equal?(x=w442, y=w441) -> (x <= y?=w439:bool)
              n256 = call "BRig_generic_convert__Prob_to_TrueFalse__boolean.vi"("input_probability_u16"=w438) -> ("output_TF"=w437:bool)  [unwired: 10 in]
              n257 = Or(x=w440, y=w439) -> (x .or. y?=w436:bool)
              n258 = And(x=w436, y=w437) -> (x .and. y?=w435:bool)
              n259 = case shown="False" w435 {
                tunnel: w434 -> [w448 _]
                tunnel: w433 -> [w447 _]
                tunnel: w432 -> [w446 _]
                tunnel: [w445 w449] -> w431
                tunnel: [w445 w451] -> w430
                tunnel: [w443 w451] -> w429
                tunnel: [u16 1 w449] -> w428
                tunnel: [w443 u16 1] -> w427
                tunnel: w426 -> [_ w454]
                tunnel: w425 -> [_ w453]
                tunnel: w424 -> [_ w452]
                frame False {
                  w443 = u16 0
                  n260 = call "BRig_generic_randomizeMinMax__v3,0.vi"("Input_Increment"=w446, "Input_Min"=w447, "Input_Max"=w448) -> ("Output"=w445:u16)  [unwired: 8 in]
                }
                frame True {
                  w449 = u16 0
                  n261 = call "BRig_generic_randomizeMinMax__v3,0.vi"("Input_Increment"=w452, "Input_Min"=w453, "Input_Max"=w454) -> ("Output"=w451:u16)  [unwired: 8 in]
                }
              }
            }
            frame 3 {
              # "Audio and LED"
              n262 = call "BRig_generic_randomizeMinMax__v3,0.vi"("Input_Increment"=w462, "Input_Min"=w463, "Input_Max"=w464) -> ("Output"=w457:u16)  [unwired: 8 in]
              n263 = call "BRig_generic_randomizeMinMax__v3,0.vi"("Input_Increment"=w459, "Input_Min"=w460, "Input_Max"=w461) -> ("Output"=w456:u16)  [unwired: 8 in]
              n264 = Greater?(x=w457, y=w456) -> (0:w458:bool)
              n265 = Select(t=w457, s=w458, f=w456) -> (s? t:f=w455:u16)
            }
          }
          n266 = call "BRig_dataTrial_sCue.vi"() -> ("output_sCue"=w350:i32)  [unwired: 11 in]
          n267 = call "BRig_dataTrial_T_Cue_Audio.vi"() -> ("output_T_Cue_Audio"=w348:i32)  [unwired: 11 in]
          n268 = call "BRig_dataTrial_T_Cue_LED.vi"() -> ("output_T_Cue_LED"=w346:i32)  [unwired: 11 in]
          n269 = call "BRig_dataCurrent_CueSwitch_Audio.vi"() -> ("output_CueSwitch_Audio"=w354:i32)  [unwired: 11 in]
          n270 = call "BRig_dataCurrent_CueSwitch_LED.vi"() -> ("output_CueSwitch_LED"=w352:i32)  [unwired: 11 in]
          n271 = call "BRig_dataCurrent_T_Cue.vi"() -> ("output_T_Cue"=w344:i32)  [unwired: 11 in]
          n272 = Replace Array Subset(array=w286, new element #1=w349, index (row) #1=w276, index (col) #1=w350, new element #2=w347, index (row) #2=w276, index (col) #2=w348, new element #3=w345, index (row) #3=w276, index (col) #3=w346) -> (w355:u16[][])
          n273 = Replace Array Subset(array=w339, new element #1=w353, index #1=w354, new element #2=w351, index #2=w352, new element #3=w343, index #3=w344) -> (w356:u16[])
        }
        frame True {
          w541 = u16 0 ("index")
          w502 = u16 0 ("new element/subarray")
          w643 = 1 ("index (row)")
          w494 = 0 ("index")
          # "T_Cue_LED"
          # "T_Cue_Audio"
          # "LED"
          # "Audio"
          # "T_Cue_LED"
          # "T_Cue_Audio"
          # "LED"
          # "Audio"
          # "Give Reward?\nL = 1A\nR = 1B"
          # "Time - Reward\nL = 1A\nR = 1B"
          # "Time - ENL2"
          # "Time - ENL1"
          # "Store last trial data into row 2\nClear row 1 for new trial data"
          n274 = call "BRig_dataCurrent_Cue2_I_1A_Sel.vi"() -> ("output_Cue2_I_1A_Sel"=w497:i32)  [unwired: 11 in]
          n275 = call "BRig_dataCurrent_Cue2_I_High_Sel.vi"() -> ("output_Cue2_I_High_Sel"=w496:i32)  [unwired: 11 in]
          n276 = call "BRig_dataCurrent_iTrial.vi"() -> ("output_iTrial"=w657:i32)  [unwired: 11 in]
          n277 = call "BRig_dataCurrent_nTrial.vi"() -> ("output_nTrial"=w578:i32)  [unwired: 11 in]
          n278 = Array Size(array=w649) -> (size(s)=w654:i32[])
          n279 = Index Array(array=w660, index #1=w497, index #2=w496, index #3=w657, index #4=w578) -> (element #1=w492:u16, element #2=w491:u16, element #3=w659:u16, element #4=w658:u16)
          n280 = Index Array(array=w654, index=1) -> (element=w652:i32)
          n281 = Index Array(array=w649, index (row)=w494) -> (element=w656:u16[])  [unwired: 1 in]
          n282 = call "BRig_dataExp_SolenoidProb_L.vi"() -> ("output_SolenoidProbability_L"=w615:i32)  [unwired: 11 in]
          n283 = call "BRig_dataExp_SolenoidProb_R.vi"() -> ("output_SolenoidProbability_R"=w616:i32)  [unwired: 11 in]
          n284 = call "BRig_dataExp_T_ENL_max.vi"() -> ("output_T_ENL_max"=w625:i32)  [unwired: 11 in]
          n285 = call "BRig_dataExp_T_ENL_min.vi"() -> ("output_T_ENL_min"=w624:i32)  [unwired: 11 in]
          n286 = call "BRig_dataExp_T_ENL_step.vi"() -> ("output_T_ENL_step"=w623:i32)  [unwired: 11 in]
          n287 = call "BRig_dataExp_T_ENL2_min.vi"() -> ("output_T_ENL2_min"=w622:i32)  [unwired: 11 in]
          n288 = call "BRig_dataExp_T_ENL2_max.vi"() -> ("output_T_ENL2_max"=w621:i32)  [unwired: 11 in]
          n289 = call "BRig_dataExp_T_ENL2_step.vi"() -> ("output_T_ENL2_step"=w620:i32)  [unwired: 11 in]
          n290 = call "BRig_dataExp_T_Reward_max_L.vi"() -> ("output_T_Reward_max_L"=w607:i32)  [unwired: 11 in]
          n291 = call "BRig_dataExp_T_Reward_max_R.vi"() -> ("output_T_Reward_max_R"=w606:i32)  [unwired: 11 in]
          n292 = call "BRig_dataExp_T_Reward_min_L.vi"() -> ("output_Tcycle_Reward_min_L"=w605:i32)  [unwired: 11 in]
          n293 = call "BRig_dataExp_T_Reward_min_R.vi"() -> ("output_T_Reward_min_R"=w604:i32)  [unwired: 11 in]
          n294 = call "BRig_dataExp_T_Reward_step_L.vi"() -> ("output_T_Reward_step_L"=w603:i32)  [unwired: 11 in]
          n295 = call "BRig_dataExp_T_Reward_step_R.vi"() -> ("output_T_Reward_step_R"=w602:i32)  [unwired: 11 in]
          n296 = call "BRig_dataExp_LaserSwitch.vi"() -> ("output_LaserSwitch"=w595:i32)  [unwired: 11 in]
          n297 = call "BRig_dataExp_LaserSwitch_Prob_l1.vi"() -> ("output_LaserSwitch_Probability_L1"=w594:i32)  [unwired: 11 in]
          n298 = call "BRig_dataExp_ClosedLoop_LaserHold_l1_I.vi"() -> ("output_CloseLoop_LaserHold_l1_I"=w593:i32)  [unwired: 11 in]
          n299 = call "BRig_dataExp_ClosedLoop_LaserHold_l2_I.vi"() -> ("output_CloseLoop_LaserHold_l2_I"=w592:i32)  [unwired: 11 in]
          n300 = Not Equal To 0?(x=w492) -> (x != 0?=w569:bool)
          n301 = Not Equal To 0?(x=w491) -> (x != 0?=w648:bool)
          n302 = Initialize Array(u16 0 ("index"), w652) -> (w650:u16[])
          n303 = Select(t=w615, s=w569, f=w616) -> (s? t:f=w614:i32)
          n304 = Select(t=w607, s=w569, f=w606) -> (s? t:f=w601:i32)
          n305 = Select(t=w605, s=w569, f=w604) -> (s? t:f=w600:i32)
          n306 = Select(t=w603, s=w569, f=w602) -> (s? t:f=w599:i32)
          n307 = Increment(x=w659) -> (x+1=w498:u16)
          n308 = Increment(x=w658) -> (x+1=w499:u16)
          n309 = call "BRig_dataTrial_Cue2_iTrial_1A.vi"() -> ("output_Cue2_iTrial_1A"=w644:i32)  [unwired: 11 in]
          n310 = call "BRig_dataTrial_Cue2_iTrial_1B.vi"() -> ("output_Cue2_iTrial_1B"=w645:i32)  [unwired: 11 in]
          n311 = call "BRig_dataTrial_Cue2_iTrial_High.vi"() -> ("output_Cue2_iTrial_High"=w647:i32)  [unwired: 11 in]
          n312 = call "BRig_dataTrial_Cue2_iTrial_Low.vi"() -> ("output_Cue2_iTrial_Low"=w646:i32)  [unwired: 11 in]
          n313 = Replace Array Subset(array=w649, new element #1=w656, index (row) #1=1 ("index (row)"), new element #2=w650, index (row) #2=w494) -> (w642:u16[][])  [unwired: 2 in]
          n314 = Select(t=w644, s=w569, f=w645) -> (s? t:f=w641:i32)
          n315 = Select(t=w647, s=w648, f=w646) -> (s? t:f=w638:i32)
          n316 = Index Array(array=w533, index #1=w614, index #2=w625, index #3=w624, index #4=w623, index #5=w622, index #6=w621, index #7=w620, index #8=w601, index #9=w600, index #10=w599, index #11=w595, index #12=w594, index #13=w593, index #14=w592) -> (element #1=w617:u16, element #2=w613:u16, element #3=w612:u16, element #4=w611:u16, element #5=w610:u16, element #6=w609:u16, element #7=w608:u16, element #8=w598:u16, element #9=w597:u16, element #10=w596:u16, element #11=w591:u16, element #12=w590:u16, element #13=w589:u16, element #14=w588:u16)
          n317 = Index Array(array=w642, index (row) #1=w643, index (col) #1=w641, index (row) #2=w643, index (col) #2=w638) -> (element #1=w640:u16, element #2=w637:u16)
          n318 = call "BRig_dataTrial_Cue2_I_1A_Sel.vi"() -> ("output_Cue2_I_1A_Sel"=w495:i32)  [unwired: 11 in]
          n319 = call "BRig_dataTrial_Cue2_I_High_Sel.vi"() -> ("output_Cue2_I_High_Sel"=w493:i32)  [unwired: 11 in]
          n320 = Increment(x=w640) -> (x+1=w639:u16)
          n321 = Increment(x=w637) -> (x+1=w636:u16)
          n322 = call "BRig_generic_convert__Prob_to_TrueFalse__boolean.vi"("input_probability_u16"=w617) -> ("output_TF"=w618:bool)  [unwired: 10 in]
          n323 = call "BRig_generic_randomizeMinMax__v3,0.vi"("Input_Increment"=w611, "Input_Min"=w612, "Input_Max"=w613) -> ("Output"=w574:u16)  [unwired: 8 in]
          n324 = call "BRig_generic_randomizeMinMax__v3,0.vi"("Input_Increment"=w608, "Input_Min"=w609, "Input_Max"=w610) -> ("Output"=w572:u16)  [unwired: 8 in]
          n325 = call "BRig_generic_randomizeMinMax__v3,0.vi"("Input_Increment"=w596, "Input_Min"=w597, "Input_Max"=w598) -> ("Output"=w570:u16)  [unwired: 8 in]
          n326 = case shown="3" w591 {
            tunnel: [w775 w776 w781 w795] -> w584
            tunnel: [w775 w777 w782 w794] -> w582
            tunnel: w590 -> [_ _ _ w798]
            tunnel: w589 -> [_ w780 _ w793]
            tunnel: w588 -> [_ _ w783 w792]
            frame 0, Default {
              w775 = u16 0
              # "No Laser"
            }
            frame 1 {
              w777 = u16 0
              # "Laser 1"
              n327 = Equal To 0?(x=w780) -> (x = 0?=w779:bool)
              n328 = Select(t=u16 1, s=w779, f=w777) -> (s? t:f=w776:u16)
            }
            frame 2 {
              w781 = u16 0
              # "Laser 2"
              n329 = Equal To 0?(x=w783) -> (x = 0?=w785:bool)
              n330 = Select(t=u16 1, s=w785, f=w781) -> (s? t:f=w782:u16)
            }
            frame 3 {
              # "Laser 1 or 2"
              n331 = Equal To 0?(x=w793) -> (x = 0?=w791:bool)
              n332 = Equal To 0?(x=w792) -> (x = 0?=w787:bool)
              n333 = call "BRig_generic_convert__Prob_to_TrueFalse__boolean.vi"("input_probability_u16"=w798) -> ("output_TF"=w790:bool)  [unwired: 10 in]
              n334 = Not(x=w790) -> (.not. x?=w788:bool)
              n335 = And(x=w787, y=w788) -> (x .and. y?=w786:bool)
              n336 = And(x=w790, y=w791) -> (x .and. y?=w789:bool)
              n337 = Boolean To (0,1)(Boolean=w786) -> (0, 1=w797:i16)
              n338 = Boolean To (0,1)(Boolean=w789) -> (0, 1=w796:i16)
              n339 = To Unsigned Word Integer(number=w797) -> (unsigned 16bit integer=w794:u16)
              n340 = To Unsigned Word Integer(number=w796) -> (unsigned 16bit integer=w795:u16)
            }
          }
          n341 = Boolean To (0,1)(Boolean=w618) -> (0, 1=w619:i16)
          n342 = Replace Array Subset(array=w660, new element #1=w498, index #1=w657, new element #2=w499, index #2=w578) -> (w587:u16[])
          n343 = Replace Array Subset(array=w642, new element #1=w639, index (row) #1=w494, index (col) #1=w641, new element #2=w636, index (row) #2=w494, index (col) #2=w638, new element #3=w492, index (row) #3=w494, index (col) #3=w495, new element #4=w491, index (row) #4=w494, index (col) #4=w493) -> (w581:u16[][])
          n344 = To Unsigned Word Integer(number=w619) -> (unsigned 16bit integer=w576:u16)
          n345 = call "BRig_dataTrial_iTrial.vi"() -> ("output_iTrial"=w580:i32)  [unwired: 11 in]
          n346 = call "BRig_dataTrial_nTrial.vi"() -> ("output_nTrial"=w579:i32)  [unwired: 11 in]
          n347 = call "BRig_dataTrial_I_giveReward.vi"() -> ("output_I_giveReward"=w577:i32)  [unwired: 11 in]
          n348 = call "BRig_dataTrial_T_ENL.vi"() -> ("output_T_ENL"=w575:i32)  [unwired: 11 in]
          n349 = call "BRig_dataTrial_T_ENL2.vi"() -> ("output_T_ENL2"=w573:i32)  [unwired: 11 in]
          n350 = call "BRig_dataTrial_T_Reward.vi"() -> ("output_T_Reward"=w571:i32)  [unwired: 11 in]
          n351 = call "BRig_dataCurrent_LaserSwitch_l1.vi"() -> ("output_LaserSwitch_l1"=w585:i32)  [unwired: 11 in]
          n352 = call "BRig_dataCurrent_LaserSwitch_l2.vi"() -> ("output_LaserSwitch_l2"=w583:i32)  [unwired: 11 in]
          n353 = Replace Array Subset(array=w581, new element #1=w498, index (row) #1=w494, index (col) #1=w580, new element #2=w499, index (row) #2=w494, index (col) #2=w579, new element #3=w576, index (row) #3=w494, index (col) #3=w577, new element #4=w574, index (row) #4=w494, index (col) #4=w575, new element #5=w572, index (row) #5=w494, index (col) #5=w573, new element #6=w570, index (row) #6=w494, index (col) #6=w571) -> (w519:u16[][])
          n354 = Replace Array Subset(array=w587, new element #1=w584, index #1=w585, new element #2=w582, index #2=w583) -> (w586:u16[])
          n355 = call "BRig_dataExp_CueSwitch_First.vi"() -> ("output_CueSwitch_First"=w568:i32)  [unwired: 11 in]
          n356 = call "BRig_dataExp_Cue2Switch_1B.vi"() -> ("output_Cue2Switch_1B"=w567:i32)  [unwired: 11 in]
          n357 = call "BRig_dataExp_CueSwitch_Prob_First.vi"() -> ("output_CueSwitch_Prob_First"=w566:i32)  [unwired: 11 in]
          n358 = call "BRig_dataExp_Cue2Switch_Prob_1B.vi"() -> ("output_Cue2Switch_Prob_1B"=w565:i32)  [unwired: 11 in]
          n359 = call "BRig_dataExp_T_Cue_Audio_max.vi"() -> ("output_T_Cue_Audio_max"=w562:i32)  [unwired: 11 in]
          n360 = call "BRig_dataExp_T_Cue_Audio_min.vi"() -> ("output_T_Cue_Audio_min"=w561:i32)  [unwired: 11 in]
          n361 = call "BRig_dataExp_T_Cue_Audio_step.vi"() -> ("output_T_Cue_Audio_step"=w560:i32)  [unwired: 11 in]
          n362 = call "BRig_dataExp_T_Cue_LED_max.vi"() -> ("output_T_Cue_LED_max"=w559:i32)  [unwired: 11 in]
          n363 = call "BRig_dataExp_T_Cue_LED_min.vi"() -> ("output_T_Cue_LED_min"=w558:i32)  [unwired: 11 in]
          n364 = call "BRig_dataExp_T_Cue_LED_step.vi"() -> ("output_T_Cue_LED_step"=w557:i32)  [unwired: 11 in]
          n365 = call "BRig_dataExp_Cue2Switch_First.vi"() -> ("output_Cue2Switch_First"=w549:i32)  [unwired: 11 in]
          n366 = call "BRig_dataExp_Cue2Switch_Prob_First.vi"() -> ("output_Cue2Switch_Prob_First"=w548:i32)  [unwired: 11 in]
          n367 = call "BRig_dataExp_T_Cue2_Audio_max.vi"() -> ("output_T_Cue2_Audio_max"=w547:i32)  [unwired: 11 in]
          n368 = call "BRig_dataExp_T_Cue2_Audio_min.vi"() -> ("output_T_Cue2_Audio_min"=w546:i32)  [unwired: 11 in]
          n369 = call "BRig_dataExp_T_Cue2_Audio_step.vi"() -> ("output_T_Cue2_Audio_step"=w545:i32)  [unwired: 11 in]
          n370 = call "BRig_dataExp_T_Cue2_LED_max.vi"() -> ("output_T_Cue2_LED_max"=w544:i32)  [unwired: 11 in]
          n371 = call "BRig_dataExp_T_Cue2_LED_min.vi"() -> ("output_T_Cue2_LED_min"=w543:i32)  [unwired: 11 in]
          n372 = call "BRig_dataExp_T_Cue2_LED_step.vi"() -> ("output_T_Cue2_LED_step"=w542:i32)  [unwired: 11 in]
          n373 = Select(t=w568, s=w569, f=w567) -> (s? t:f=w564:i32)
          n374 = Select(t=w566, s=w569, f=w565) -> (s? t:f=w563:i32)
          n375 = call "BRig_dataCurrent_t_selection.vi"() -> ("output_t_selection"=w635:i32)  [unwired: 11 in]
          n376 = call "BRig_dataCurrent_s_Selection.vi"() -> ("output_s_Selection"=w634:i32)  [unwired: 11 in]
          n377 = call "BRig_dataCurrent_I_anySelect_L.vi"() -> ("output_IanySelect_L"=w633:i32)  [unwired: 11 in]
          n378 = call "BRig_dataCurrent_I_anySelect_R.vi"() -> ("output_IanySelect_R"=w632:i32)  [unwired: 11 in]
          n379 = call "BRig_dataCurrent_L_ENL_I_l1.vi"() -> ("output_L_ENL_I_l1"=w631:i32)  [unwired: 11 in]
          n380 = call "BRig_dataCurrent_L_ENL_I_l2.vi"() -> ("output_L_ENL_I_l2"=w630:i32)  [unwired: 11 in]
          n381 = call "BRig_dataCurrent_L_Cue_I_l1.vi"() -> ("output_L_Cue_I_l1"=w629:i32)  [unwired: 11 in]
          n382 = call "BRig_dataCurrent_L_Cue_I_l2.vi"() -> ("output_L_Cue_I_l2"=w628:i32)  [unwired: 11 in]
          n383 = call "BRig_dataCurrent_L_Sel_I_l1.vi"() -> ("output_L_Sel_I_l1"=w627:i32)  [unwired: 11 in]
          n384 = call "BRig_dataCurrent_L_Sel_I_l2.vi"() -> ("output_L_Sel_I_l2"=w626:i32)  [unwired: 11 in]
          n385 = Index Array(array=w533, index #1=w564, index #2=w563, index #3=w562, index #4=w561, index #5=w560, index #6=w559, index #7=w558, index #8=w557, index #9=w549, index #10=w548, index #11=w547, index #12=w546, index #13=w545, index #14=w544, index #15=w543, index #16=w542) -> (element #1=w518:u16, element #2=w556:u16, element #3=w555:u16, element #4=w554:u16, element #5=w553:u16, element #6=w552:u16, element #7=w551:u16, element #8=w550:u16, element #9=w512:u16, element #10=w540:u16, element #11=w539:u16, element #12=w538:u16, element #13=w537:u16, element #14=w536:u16, element #15=w535:u16, element #16=w534:u16)
          n386 = call "BRig_dataCurrent_L_ENL2_I_l1.vi"() -> ("output_L_ENL2_I_l1"=w506:i32)  [unwired: 11 in]
          n387 = call "BRig_dataCurrent_L_ENL2_I_l2.vi"() -> ("output_L_ENL2_I_l2"=w505:i32)  [unwired: 11 in]
          n388 = call "BRig_dataCurrent_L_Cue2_I_l1.vi"() -> ("output_L_Cue2_I_l1"=w504:i32)  [unwired: 11 in]
          n389 = call "BRig_dataCurrent_L_Cue2_I_l2.vi"() -> ("output_L_Cue2_I_l2"=w503:i32)  [unwired: 11 in]
          n390 = Replace Array Subset(array=w586, new element #1=w502, index #1=w635, new element #2=w502, index #2=w634, new element #3=w502, index #3=w633, new element #4=w502, index #4=w632, new element #5=w502, index #5=w631, new element #6=w502, index #6=w630, new element #7=w502, index #7=w629, new element #8=w502, index #8=w628, new element #9=w502, index #9=w627, new element #10=w502, index #10=w626, new element #11=w502, index #11=w506, new element #12=w502, index #12=w505, new element #13=w502, index #13=w504, new element #14=w502, index #14=w503) -> (w520:u16[])
          n391 = case shown="2" w518 {
            tunnel: [u16 1 u16 0 w736 u16 1] -> w531
            tunnel: [u16 0 u16 1 w735 u16 1] -> w529
            tunnel: w541 -> [_ _ w749 _]
            tunnel: w556 -> [_ _ w746 _]
            tunnel: w555 -> [w722 _ w742 w772]
            tunnel: w554 -> [w721 _ w741 w771]
            tunnel: w553 -> [w720 _ w740 w770]
            tunnel: w552 -> [_ w729 w734 w769]
            tunnel: w551 -> [_ w728 w733 w768]
            tunnel: w550 -> [_ w727 w732 w767]
            tunnel: [w719 u16 0 ("Output") w739 w765] -> w515
            tunnel: [u16 0 ("Output") w726 w737 w764] -> w513
            tunnel: [w719 w726 w738 w763] -> w527
            tunnel: w541 -> [_ _ w750 _]
            frame 0, Default {
              # "Audio only"
              n392 = call "BRig_generic_randomizeMinMax__v3,0.vi"("Input_Increment"=w720, "Input_Min"=w721, "Input_Max"=w722) -> ("Output"=w719:u16)  [unwired: 8 in]
            }
            frame 1 {
              # "LED only"
              n393 = call "BRig_generic_randomizeMinMax__v3,0.vi"("Input_Increment"=w727, "Input_Min"=w728, "Input_Max"=w729) -> ("Output"=w726:u16)  [unwired: 8 in]
            }
            frame 2 {
              # "Audio or LED"
              n394 = Equal To 0?(x=w750) -> (x = 0?=w748:bool)
              n395 = Less Or Equal?(x=w750, y=w749) -> (x <= y?=w747:bool)
              n396 = call "BRig_generic_convert__Prob_to_TrueFalse__boolean.vi"("input_probability_u16"=w746) -> ("output_TF"=w745:bool)  [unwired: 10 in]
              n397 = Or(x=w748, y=w747) -> (x .or. y?=w744:bool)
              n398 = And(x=w744, y=w745) -> (x .and. y?=w743:bool)
              n399 = case shown="False" w743 {
                tunnel: w742 -> [w756 _]
                tunnel: w741 -> [w755 _]
                tunnel: w740 -> [w754 _]
                tunnel: [w753 w757] -> w739
                tunnel: [w753 w759] -> w738
                tunnel: [w751 w759] -> w737
                tunnel: [u16 1 w757] -> w736
                tunnel: [w751 u16 1] -> w735
                tunnel: w734 -> [_ w762]
                tunnel: w733 -> [_ w761]
                tunnel: w732 -> [_ w760]
                frame False {
                  w751 = u16 0
                  n400 = call "BRig_generic_randomizeMinMax__v3,0.vi"("Input_Increment"=w754, "Input_Min"=w755, "Input_Max"=w756) -> ("Output"=w753:u16)  [unwired: 8 in]
                }
                frame True {
                  w757 = u16 0
                  n401 = call "BRig_generic_randomizeMinMax__v3,0.vi"("Input_Increment"=w760, "Input_Min"=w761, "Input_Max"=w762) -> ("Output"=w759:u16)  [unwired: 8 in]
                }
              }
            }
            frame 3 {
              # "Audio and LED"
              n402 = call "BRig_generic_randomizeMinMax__v3,0.vi"("Input_Increment"=w770, "Input_Min"=w771, "Input_Max"=w772) -> ("Output"=w765:u16)  [unwired: 8 in]
              n403 = call "BRig_generic_randomizeMinMax__v3,0.vi"("Input_Increment"=w767, "Input_Min"=w768, "Input_Max"=w769) -> ("Output"=w764:u16)  [unwired: 8 in]
              n404 = Greater?(x=w765, y=w764) -> (0:w766:bool)
              n405 = Select(t=w765, s=w766, f=w764) -> (s? t:f=w763:u16)
            }
          }
          n406 = case shown="2" w512 {
            tunnel: [u16 1 u16 0 w679 u16 1] -> w525
            tunnel: [u16 0 u16 1 w678 u16 1] -> w523
            tunnel: w541 -> [_ _ w692 _]
            tunnel: w540 -> [_ _ w689 _]
            tunnel: w539 -> [w665 _ w685 w715]
            tunnel: w538 -> [w664 _ w684 w714]
            tunnel: w537 -> [w663 _ w683 w713]
            tunnel: w536 -> [_ w672 w677 w712]
            tunnel: w535 -> [_ w671 w676 w711]
            tunnel: w534 -> [_ w670 w675 w710]
            tunnel: [w662 u16 0 ("Output") w682 w708] -> w509
            tunnel: [u16 0 ("Output") w669 w680 w707] -> w507
            tunnel: [w662 w669 w681 w706] -> w521
            tunnel: w541 -> [_ _ w693 _]
            frame 0, Default {
              # "Audio only"
              n407 = call "BRig_generic_randomizeMinMax__v3,0.vi"("Input_Increment"=w663, "Input_Min"=w664, "Input_Max"=w665) -> ("Output"=w662:u16)  [unwired: 8 in]
            }
            frame 1 {
              # "LED only"
              n408 = call "BRig_generic_randomizeMinMax__v3,0.vi"("Input_Increment"=w670, "Input_Min"=w671, "Input_Max"=w672) -> ("Output"=w669:u16)  [unwired: 8 in]
            }
            frame 2 {
              # "Audio or LED"
              n409 = Equal To 0?(x=w693) -> (x = 0?=w691:bool)
              n410 = Less Or Equal?(x=w693, y=w692) -> (x <= y?=w690:bool)
              n411 = call "BRig_generic_convert__Prob_to_TrueFalse__boolean.vi"("input_probability_u16"=w689) -> ("output_TF"=w688:bool)  [unwired: 10 in]
              n412 = Or(x=w691, y=w690) -> (x .or. y?=w687:bool)
              n413 = And(x=w687, y=w688) -> (x .and. y?=w686:bool)
              n414 = case shown="False" w686 {
                tunnel: w685 -> [w699 _]
                tunnel: w684 -> [w698 _]
                tunnel: w683 -> [w697 _]
                tunnel: [w696 w700] -> w682
                tunnel: [w696 w702] -> w681
                tunnel: [w694 w702] -> w680
                tunnel: [u16 1 w700] -> w679
                tunnel: [w694 u16 1] -> w678
                tunnel: w677 -> [_ w705]
                tunnel: w676 -> [_ w704]
                tunnel: w675 -> [_ w703]
                frame False {
                  w694 = u16 0
                  n415 = call "BRig_generic_randomizeMinMax__v3,0.vi"("Input_Increment"=w697, "Input_Min"=w698, "Input_Max"=w699) -> ("Output"=w696:u16)  [unwired: 8 in]
                }
                frame True {
                  w700 = u16 0
                  n416 = call "BRig_generic_randomizeMinMax__v3,0.vi"("Input_Increment"=w703, "Input_Min"=w704, "Input_Max"=w705) -> ("Output"=w702:u16)  [unwired: 8 in]
                }
              }
            }
            frame 3 {
              # "Audio and LED"
              n417 = call "BRig_generic_randomizeMinMax__v3,0.vi"("Input_Increment"=w713, "Input_Min"=w714, "Input_Max"=w715) -> ("Output"=w708:u16)  [unwired: 8 in]
              n418 = call "BRig_generic_randomizeMinMax__v3,0.vi"("Input_Increment"=w710, "Input_Min"=w711, "Input_Max"=w712) -> ("Output"=w707:u16)  [unwired: 8 in]
              n419 = Greater?(x=w708, y=w707) -> (0:w709:bool)
              n420 = Select(t=w708, s=w709, f=w707) -> (s? t:f=w706:u16)
            }
          }
          n421 = call "BRig_dataTrial_sCue.vi"() -> ("output_sCue"=w517:i32)  [unwired: 11 in]
          n422 = call "BRig_dataCurrent_CueSwitch_Audio.vi"() -> ("output_CueSwitch_Audio"=w532:i32)  [unwired: 11 in]
          n423 = call "BRig_dataCurrent_CueSwitch_LED.vi"() -> ("output_CueSwitch_LED"=w530:i32)  [unwired: 11 in]
          n424 = call "BRig_dataTrial_T_Cue_Audio.vi"() -> ("output_T_Cue_Audio"=w516:i32)  [unwired: 11 in]
          n425 = call "BRig_dataTrial_T_Cue_LED.vi"() -> ("output_T_Cue_LED"=w514:i32)  [unwired: 11 in]
          n426 = call "BRig_dataCurrent_T_Cue.vi"() -> ("output_T_Cue"=w528:i32)  [unwired: 11 in]
          n427 = call "BRig_dataTrial_sCue2.vi"() -> ("output_sCue2"=w511:i32)  [unwired: 11 in]
          n428 = call "BRig_dataCurrent_Cue2Switch_Audio.vi"() -> ("output_Cue2Switch_Audio"=w526:i32)  [unwired: 11 in]
          n429 = call "BRig_dataCurrent_Cue2Switch_LED.vi"() -> ("output_Cue2Switch_LED"=w524:i32)  [unwired: 11 in]
          n430 = call "BRig_dataTrial_T_Cue2_Audio.vi"() -> ("output_T_Cue2_Audio"=w510:i32)  [unwired: 11 in]
          n431 = call "BRig_dataTrial_T_Cue2_LED.vi"() -> ("output_T_Cue2_LED"=w508:i32)  [unwired: 11 in]
          n432 = call "BRig_dataCurrent_T_Cue2.vi"() -> ("output_T_Cue2"=w522:i32)  [unwired: 11 in]
          n433 = Replace Array Subset(array=w520, new element #1=w531, index #1=w532, new element #2=w529, index #2=w530, new element #3=w527, index #3=w528, new element #4=w525, index #4=w526, new element #5=w523, index #5=w524, new element #6=w521, index #6=w522) -> (w501:u16[])
          n434 = Replace Array Subset(array=w519, new element #1=w518, index (row) #1=w494, index (col) #1=w517, new element #2=w515, index (row) #2=w494, index (col) #2=w516, new element #3=w513, index (row) #3=w494, index (col) #3=w514, new element #4=w512, index (row) #4=w494, index (col) #4=w511, new element #5=w509, index (row) #5=w494, index (col) #5=w510, new element #6=w507, index (row) #6=w494, index (col) #6=w508) -> (w500:u16[][])
        }
      }
    }
  }
  "output_dataBlock" <- w14
  "output_dataTrial" <- w13
  "output_dataCurrent" <- w12
  "output_SolenoidReward" <- w11
  "output_nTrial" <- w10
  "output_iTrial" <- w9
